vi "单参数加标流程.vi"(10 "流程类型":T4, 11 "Slave ID":T6=enum."氨氮") -> ()   [LabVIEW 2016, in "质控单元V1.lvlib"]
panel:
  in  "平行样测试数据":T1={"时间"=timestamp(0 s since 1904-01-01), "参数"="", "数据类型"="N", "第一次水样浓度值"=0.0, "第二次水样测试时间"=timestamp(0 s since 1904-01-01), "第二次水样浓度值"=0.0}
  in  "集成干预测试数据":T2={"时间"=timestamp(0 s since 1904-01-01), "参数"="", "数据类型"="N", "集成干预测试浓度值"=0.0, "集成干预前测试时间"=timestamp(0 s since 1904-01-01), "集成干预前测试浓度值"=0.0}
  out "平行样启动时间":timestamp
  out "加标模块润洗流程控制":T3=enum."排液"
  in  "获取加标回收测试数据计数":u16
  in  "获取水样测试数据计数":u16
  in  "写入加标体积重试次数":u16
  in  "加标模块加标润洗启动计数":u16
  out "加标回收启动时间":timestamp
  out "水样测试启动时间":timestamp
  out "Next State":string
  in  "仪器加标回收启动计数":u16
  in  "仪器水样测试启动计数":u16
  in  "加标模块排液启动计数":u16
  in  "加标模块加标启动计数":u16
  in  "加标模块进样启动计数":u16
  in  "加标模块水样润洗启动计数":u16
  in  "采配水启动次数计数":u16
  in  "加标回收测试时间":timestamp
  in  "水样测试时间":timestamp
  in  "质控数据":T5
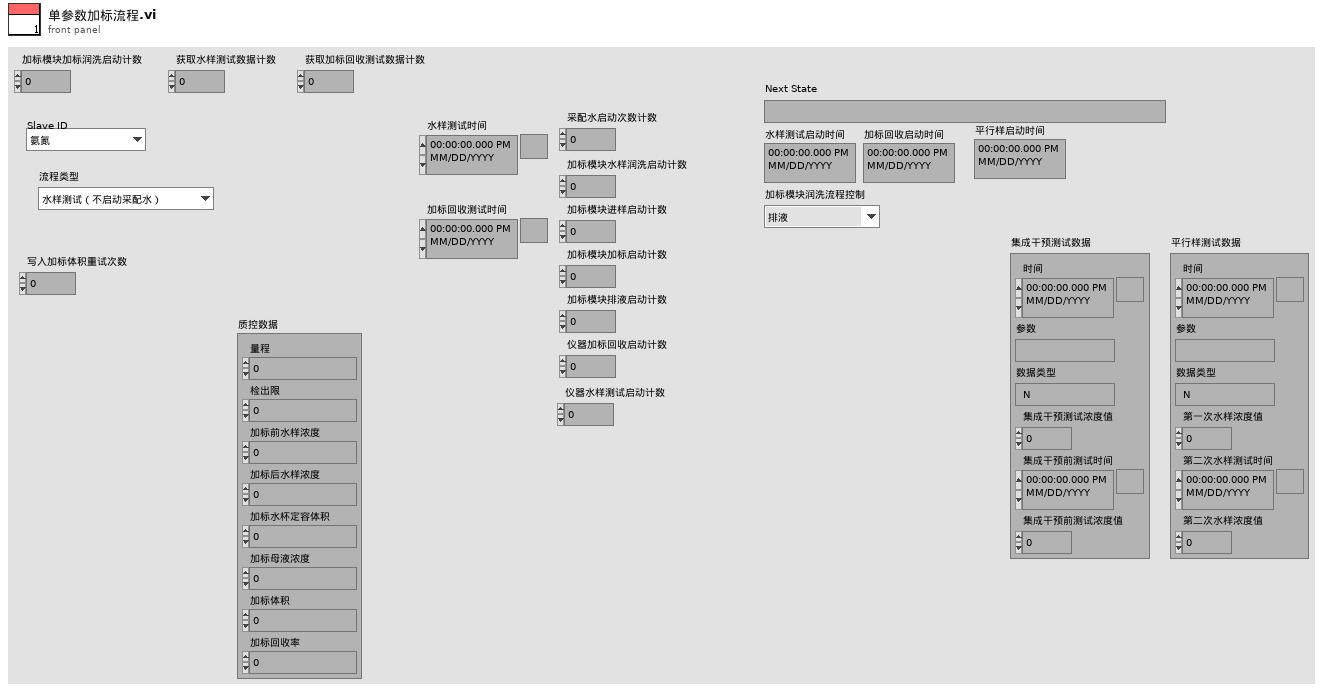
[diagram p1: front panel]
types:
  T1 = typedef "平行样测试数据字段定义.ctl" = cluster{"时间":timestamp, "参数":string, "数据类型":string, "第一次水样浓度值":dbl, "第二次水样测试时间":timestamp, "第二次水样浓度值":dbl}
  T2 = typedef "集成干预字段定义.ctl" = cluster{"时间":timestamp, "参数":string, "数据类型":string, "集成干预测试浓度值":dbl, "集成干预前测试时间":timestamp, "集成干预前测试浓度值":dbl}
  T3 = typedef "质控单元V1.lvlib/质控流程控制.ctl" = enum16{"待机", "润洗", "进样", "加标", "排液", "搅拌"}
  T4 = typedef "质控单元V1.lvlib/测试子流程.ctl" = enum16{"水样测试（不启动采配水）", "水样测试（不含采样杯）", "加标回收（润洗采样合并）", "加标回收（不启动采配水）", "平行样测试（不启动采配水）", "平行样测试（不含采样杯）", "集成干预测试（不含采样杯）"}
  T5 = cluster{"量程":dbl, "检出限":dbl, "加标前水样浓度":dbl, "加标后水样浓度":dbl, "加标水杯定容体积":dbl, "加标母液浓度":dbl, "加标体积":dbl, "加标回收率":dbl}
  T6 = typedef "质控单元V1.lvlib/质控slave id.ctl" = enum16{"null", "氨氮", "总磷", "CODMn", "CODCr", "总氮"}
  T7 = cluster{"时间":timestamp, "参数":string, "数据类型":string, "加标回收率":sgl, "加标前水样测试时间":timestamp, "加标前水样浓度值":sgl, "加标后水样浓度值":sgl, "加标母液浓度值":sgl, "加标体积":sgl, "加标水杯定容体积":sgl}
  T8 = enum16{"待机", "水样测试（全流程）", "停止", "加标回收", "水样测试（简易流程）"}
  T9 = enum16{"待机", "润洗", "采样", "沉淀", "配水", "反冲洗", "储水", "结束"}
  T10 = typedef "质控单元V1.lvlib/采配水通用流程.ctl" = enum16{"待机", "润洗", "采样", "沉淀", "配水", "反冲洗", "结束"}
  T11 = typedef "质控单元V1.lvlib/质控运行状态.ctl" = enum16{"待机", "润洗", "进样", "加标", "排液", "搅拌", "超时告警"}
  T12 = enum16{"空闲", "水样测试", "标样核查", "零点核查", "跨度核查", "空白测试", "平行样测试", "加标回收", "空白校准", "标样校准", "初始化（清洗）"}
  T13 = cluster{"时间":timestamp, "参数":string, "数据类型":string, "第一次水样浓度值":dbl, "第二次水样测试时间":timestamp, "第二次水样浓度值":dbl}
  T14 = cluster{"水样数据时间":timestamp, "水样实测值":sgl, "水样数据标识":string}
  T15 = cluster{"加标回收数据时间":timestamp, "加标回收实测值":sgl, "加标回收数据标识":string}
  T16 = typedef "质控单元V1.lvlib/质控仪器状态.ctl" = cluster{"运行状态":T11, "加标体积":sgl, "NC":dbl, "液位状态":enum16{"无感应", "有感应"}, "告警状态":enum16{"无告警", "超时告警"}}
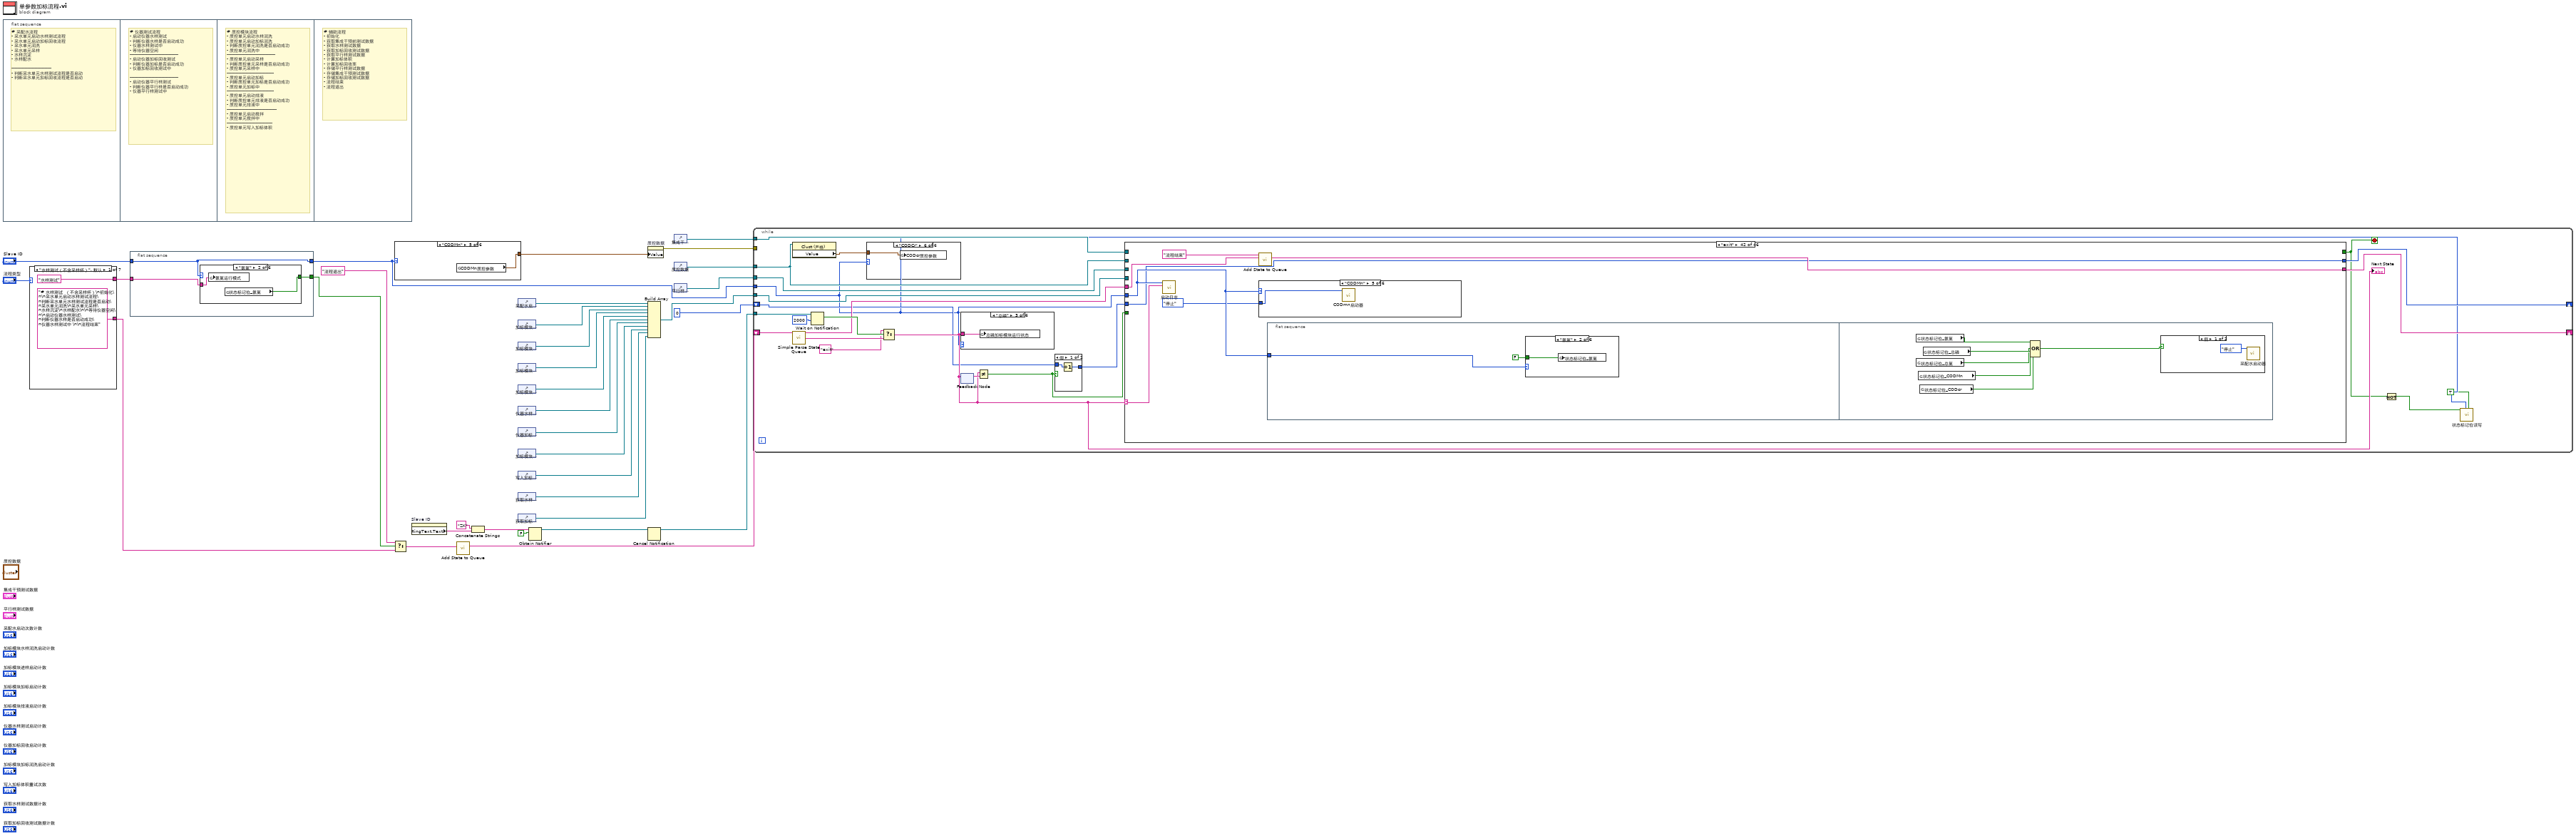
[diagram p0: block diagram]
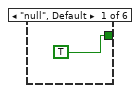
[diagram p2: hidden frame]
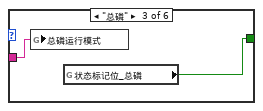
[diagram p3: hidden frame]
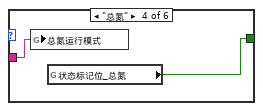
[diagram p4: hidden frame]
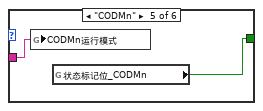
[diagram p5: hidden frame]
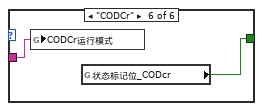
[diagram p6: hidden frame]
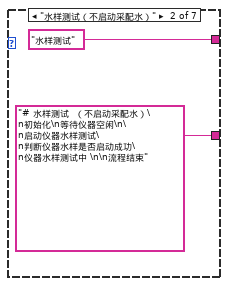
[diagram p7: hidden frame]
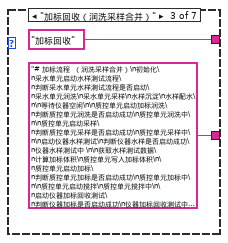
[diagram p8: hidden frame]
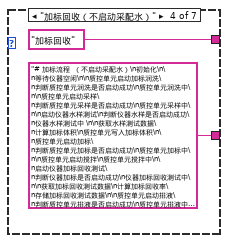
[diagram p9: hidden frame]
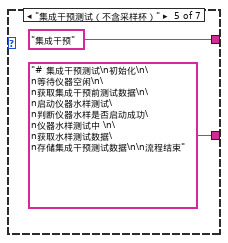
[diagram p10: hidden frame]
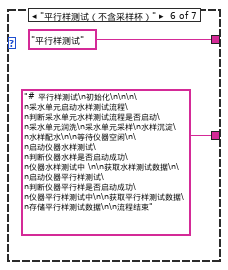
[diagram p11: hidden frame]
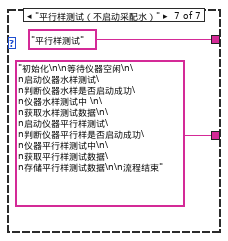
[diagram p12: hidden frame]
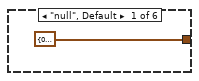
[diagram p13: hidden frame]
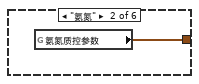
[diagram p14: hidden frame]
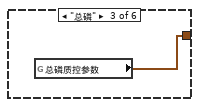
[diagram p15: hidden frame]
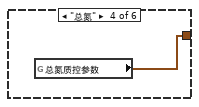
[diagram p16: hidden frame]
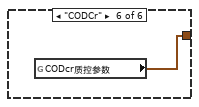
[diagram p17: hidden frame]
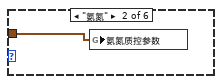
[diagram p20: hidden frame]
diagram:
  n1 = flat-sequence {
    frame #0 {
      # "# 采配水流程\n- 采水单元启动水样测试流程\n- 采水单元启动加标回收流程\n- 采水单元润洗\n- 采水单元采样 \n- 水样沉淀\n- 水样配水\n\n----------------------------\n- 判断采水单元水样测试流程是否启动\n- 判断采水单元加标回收流程是否启动"
    }
    frame #1 {
      # "# 仪器测试流程\n- 启动仪器水样测试\n- 判断仪器水样是否启动成功\n- 仪器水样测试中\n- 等待仪器空闲\n----------------------------------\n- 启动仪器加标回收测试\n- 判断仪器加标是否启动成功\n- 仪器加标回收测试中\n\n----------------------------------\n- 启动仪器平行样测试\n- 判断仪器平行样是否启动成功\n- 仪器平行样测试中"
    }
    frame #2 {
      # "# 质控模块流程\n- 质控单元启动水样润洗\n- 质控单元启动加标润洗\n- 判断质控单元润洗是否启动成功\n- 质控单元润洗中\n----------------------------------\n- 质控单元启动采样\n- 判断质控单元采样是否启动成功\n- 质控单元采样中\n---------------------------------\n- 质控单元启动加标\n- 判断质控单元加标是否启动成功\n- 质控单元加标中\n---------------------------------\n- 质控单元启动排液\n- 判断质控单元排液是否启动成功\n- 质控单元排液中\n-----------------------------------\n- 质控单元启动搅拌\n- 质控单元搅拌中\n--------------------------------\n- 质控单元写入加标体积"
    }
    frame #3 {
      # "# 辅助流程\n- 初始化\n- 获取集成干预前测试数据\n- 获取水样测试数据\n- 获取加标回收测试数据\n- 获取平行样测试数据\n- 计算加标体积\n- 计算加标回收率\n- 存储平行样测试数据\n- 存储集成干预测试数据\n- 存储加标回收测试数据 \n- 流程结束\n- 流程退出"
    }
  }
  n2 = case shown="\"水样测试（不含采样杯）\", 默认" "流程类型" {
    tunnel: ["# 水样测试  （不含采样杯）\n初始化\n\n采水单元启动水样测试流程\n判断采水单元水样测试流程是否启动\n采水单元润洗\n采水单元采样\n水样沉淀\n水样配水\n\n等待仪器空闲\n\n启动仪器水样测试\n判断仪器水样是否启动成功\n仪器水样测试中 \n\n流程结束" ("State(s) In (\"\")") "# 水样测试  （不启动采配水）\n初始化\n等待仪器空闲\n\n启动仪器水样测试\n判断仪器水样是否启动成功\n仪器水样测试中 \n\n流程结束" ("State(s) In (\"\")") "# 加标流程  （润洗采样合并）\n初始化\n采水单元启动水样测试流程\n判断采水单元水样测试流程是否启动\n采水单元润洗\n采水单元采样\n水样沉淀\n水样配水\n\n等待仪器空闲\n\n质控单元启动加标润洗\n判断质控单元润洗是否启动成功\n质控单元润洗中\n\n质控单元启动采样\n判断质控单元采样是否启动成功\n质控单元采样中\n\n启动仪器水样测试\n判断仪器水样是否启动成功\n仪器水样测试中 \n\n获取水样测试数据\n计算加标体积\n质控单元写入加标体积\n\n质控单元启动加标\n判断质控单元加标是否启动成功\n质控单元加标中\n\n质控单元启动搅拌\n质控单元搅拌中\n\n启动仪器加标回收测试\n判断仪器加标是否启动成功\n仪器加标回收测试中\n\n获取加标回收测试数据\n计算加标回收率\n存储加标回收测试数据\n\n质控单元启动排液\n判断质控单元排液是否启动成功\n质控单元排液中\n\n流程结束" ("State(s) In (\"\")") "# 加标流程  （不启动采配水）\n初始化\n\n等待仪器空闲\n\n质控单元启动加标润洗\n判断质控单元润洗是否启动成功\n质控单元润洗中\n\n质控单元启动采样\n判断质控单元采样是否启动成功\n质控单元采样中\n\n启动仪器水样测试\n判断仪器水样是否启动成功\n仪器水样测试中 \n\n获取水样测试数据\n计算加标体积\n质控单元写入加标体积\n\n质控单元启动加标\n判断质控单元加标是否启动成功\n质控单元加标中\n\n质控单元启动搅拌\n质控单元搅拌中\n\n启动仪器加标回收测试\n判断仪器加标是否启动成功\n仪器加标回收测试中\n\n获取加标回收测试数据\n计算加标回收率\n存储加标回收测试数据\n\n质控单元启动排液\n判断质控单元排液是否启动成功\n质控单元排液中\n\n流程结束" ("State(s) In (\"\")") "# 集成干预测试\n初始化\n\n等待仪器空闲\n\n获取集成干预前测试数据\n\n启动仪器水样测试\n判断仪器水样是否启动成功\n仪器水样测试中 \n\n获取水样测试数据\n存储集成干预测试数据\n\n流程结束" ("State(s) In (\"\")") "# 平行样测试\n初始化\n\n\n\n采水单元启动水样测试流程\n判断采水单元水样测试流程是否启动\n采水单元润洗\n采水单元采样\n水样沉淀\n水样配水\n\n等待仪器空闲\n\n启动仪器水样测试\n判断仪器水样是否启动成功\n仪器水样测试中 \n\n获取水样测试数据\n\n启动仪器平行样测试\n判断仪器平行样是否启动成功\n仪器平行样测试中\n\n获取平行样测试数据\n存储平行样测试数据\n\n流程结束" ("State(s) In (\"\")") "初始化\n\n等待仪器空闲\n\n启动仪器水样测试\n判断仪器水样是否启动成功\n仪器水样测试中 \n\n获取水样测试数据\n\n启动仪器平行样测试\n判断仪器平行样是否启动成功\n仪器平行样测试中\n\n获取平行样测试数据\n存储平行样测试数据\n\n流程结束" ("State(s) In (\"\")")] -> w12
    tunnel: ["水样测试" "水样测试" "加标回收" "加标回收" "集成干预" "平行样测试" "平行样测试"] -> w6
    frame "水样测试（不含采样杯）", Default {
    }
    frame "水样测试（不启动采配水）" {
    }
    frame "加标回收（润洗采样合并）" {
    }
    frame "加标回收（不启动采配水）" {
    }
    frame "集成干预测试（不含采样杯）" {
    }
    frame "平行样测试（不含采样杯）" {
    }
    frame "平行样测试（不启动采配水）" {
    }
  }
  n3 = flat-sequence {
    tunnel: [w49] -> w15
    tunnel: [w50] -> w14
    tunnel: "Slave ID" -> [w49]
    tunnel: w6 -> [w48]
    frame #0 {
      n4 = case shown="\"氨氮\"" w49 {
        tunnel: [TRUE w52 w54 w56 w58 w60] -> w50
        tunnel: w48 -> [_ w53 w55 w57 w59 w61]
        frame "null", Default {
        }
        frame "氨氮" {
          n5 = global write "ZK非断电保存全局变量.vi" "氨氮运行模式"(w53) -> ()
          n6 = global read "ZK非断电保存全局变量.vi" "状态标记位_氨氮"() -> (w52:bool)
        }
        frame "总磷" {
          n7 = global write "ZK非断电保存全局变量.vi" "总磷运行模式"(w55) -> ()
          n8 = global read "ZK非断电保存全局变量.vi" "状态标记位_总磷"() -> (w54:bool)
        }
        frame "总氮" {
          n9 = global write "ZK非断电保存全局变量.vi" "总氮运行模式"(w57) -> ()
          n10 = global read "ZK非断电保存全局变量.vi" "状态标记位_总氮"() -> (w56:bool)
        }
        frame "CODMn" {
          n11 = global write "ZK非断电保存全局变量.vi" "CODMn运行模式"(w59) -> ()
          n12 = global read "ZK非断电保存全局变量.vi" "状态标记位_CODMn"() -> (w58:bool)
        }
        frame "CODCr" {
          n13 = global write "ZK非断电保存全局变量.vi" "CODCr运行模式"(w61) -> ()
          n14 = global read "ZK非断电保存全局变量.vi" "状态标记位_CODcr"() -> (w60:bool)
        }
      }
    }
  }
  n15 = Select(t="流程退出", s=w14, f=w12) -> (s? t:f=w11:string)
  n16 = case shown="\"CODMn\"" w15 {
    tunnel: [T5 {"量程"=0.0, "检出限"=0.0, "加标前水样浓度"=0.0, "加标后水样浓度"=0.0, "加标水杯定容体积"=0.0, "加标母液浓度"=0.0, "加标体积"=0.0, "加标回收率"=0.0} ("CODcr质控参数") w63 w64 w65 w66 w67] -> w25
    frame "null", Default {
    }
    frame "氨氮" {
      n17 = global read "ZK断电保存全局变量.vi" "氨氮质控参数"() -> (w63:T5)
    }
    frame "总磷" {
      n18 = global read "ZK断电保存全局变量.vi" "总磷质控参数"() -> (w64:T5)
    }
    frame "总氮" {
      n19 = global read "ZK断电保存全局变量.vi" "总氮质控参数"() -> (w65:T5)
    }
    frame "CODMn" {
      n20 = global read "ZK断电保存全局变量.vi" "CODMn质控参数"() -> (w66:T5)
    }
    frame "CODCr" {
      n21 = global read "ZK断电保存全局变量.vi" "CODcr质控参数"() -> (w67:T5)
    }
  }
  n22 = property on="Slave ID" class="Enum (严格)"() -> ("RingText.Text"=w33:string)  [unwired: 2 in, 2 out]
  n23 = call "Add State to Queue.vi"("State(s) In (\"\")"=w11) -> ("States Out"=w27:string)  [unwired: 14 in]
  n24 = Concatenate Strings("ZK" ("字符串"), w33) -> (w31:string)
  n25 = control-ref of="采配水启动次数计数"() -> (w23:refnum<vi>)
  n26 = control-ref of="加标模块水样润洗启动计数"() -> (w22:refnum<vi>)
  n27 = control-ref of="加标模块进样启动计数"() -> (w21:refnum<vi>)
  n28 = control-ref of="加标模块加标启动计数"() -> (w20:refnum<vi>)
  n29 = control-ref of="加标模块排液启动计数"() -> (w19:refnum<vi>)
  n30 = control-ref of="仪器水样测试启动计数"() -> (w4:refnum<vi>)
  n31 = control-ref of="仪器加标回收启动计数"() -> (w5:refnum<vi>)
  n32 = control-ref of="加标模块加标润洗启动计数"() -> (w16:refnum<vi>)
  n33 = control-ref of="写入加标体积重试次数"() -> (w10:refnum<vi>)
  n34 = control-ref of="获取水样测试数据计数"() -> (w9:refnum<vi>)
  n35 = control-ref of="获取加标回收测试数据计数"() -> (w8:refnum<vi>)
  n36 = Obtain Notifier(name (unnamed)=w31, notification data type=FALSE) -> (notifier out=w29:refnum<notifier>)  [unwired: 2 in, 2 out]
  n37 = property on="质控数据" class="Clust (严格)"("Value"=w25) -> (error out=w26:errorcluster)  [unwired: 2 in, 1 out]
  n38 = Build Array(w23, w22, w21, w20, w19, w4, w5, w16, w10, w9, w8) -> (w18:refnum<vi>[])
  n39 = Cancel Notification(0:w29) -> (8:w28:refnum<notifier>)  [unwired: 1 in, 2 out]
  n40 = control-ref of="集成干预测试数据"() -> (w2:refnum<vi>)
  n41 = control-ref of="质控数据"() -> (w24:refnum<vi>)
  n42 = control-ref of="平行样测试数据"() -> (w1:refnum<vi>)
  n43 = while {
    tunnel: w28 -> [w89]
    tunnel: w15 -> [w69]
    shift-right: [w83] -> _
    shift-left: w27 -> [w90]
    tunnel: w26 -> [_]
    tunnel: w24 -> [w82]
    tunnel: w18 -> [w80]
    shift-right: [w75] -> _
    shift-left: 0 -> [w77]
    tunnel: w2 -> [w72]
    tunnel: w1 -> [w73]
    stop <- w71 stop-if-true
    n44 = property class="Clust (严格)"(reference=w82) -> ("Value"=w81:T5)  [unwired: 1 in, 2 out]
    n45 = call "Simple Parse State Queue.vi"("State Queue"=w90) -> ("Remain States"=w84:string, "Next State"=w86:string)  [unwired: 13 in]
    n46 = Wait on Notification(notifier=w89, timeout in ms (-1)=2000 ("超时毫秒(-1)")) -> (notification=w87:bool)  [unwired: 2 in, 3 out]
    n47 = case shown="\"CODCr\"" w69 {
      tunnel: w81 -> [_ w93 w94 w95 w96 w97]
      frame "null", Default {
      }
      frame "氨氮" {
        n48 = global write "ZK断电保存全局变量.vi" "氨氮质控参数"(w93) -> ()
      }
      frame "总磷" {
        n49 = global write "ZK断电保存全局变量.vi" "总磷质控参数"(w94) -> ()
      }
      frame "总氮" {
        n50 = global write "ZK断电保存全局变量.vi" "总氮质控参数"(w95) -> ()
      }
      frame "CODMn" {
        n51 = global write "ZK断电保存全局变量.vi" "CODMn质控参数"(w96) -> ()
      }
      frame "CODCr" {
        n52 = global write "ZK断电保存全局变量.vi" "CODcr质控参数"(w97) -> ()
      }
    }
    n53 = Select(t="exit" ("State(s) In (\"\")"), s=w87, f=w86) -> (s? t:f=w78:string)
    "Next State" <- w78
    n54 = case shown="\"总磷\"" w69 {
      tunnel: w78 -> [_ w98 w99 w100 w101 w102]
      frame "null", Default {
      }
      frame "氨氮" {
        n55 = global write "ZK非断电保存全局变量.vi" "氨氮加标模块运行状态"(w98) -> ()
      }
      frame "总磷" {
        n56 = global write "ZK非断电保存全局变量.vi" "总磷加标模块运行状态"(w99) -> ()
      }
      frame "总氮" {
        n57 = global write "ZK非断电保存全局变量.vi" "总氮加标模块运行状态"(w100) -> ()
      }
      frame "CODMn" {
        n58 = global write "ZK非断电保存全局变量.vi" "CODMn加标模块运行状态"(w101) -> ()
      }
      frame "CODCr" {
        n59 = global write "ZK非断电保存全局变量.vi" "CODcr加标模块运行状态"(w102) -> ()
      }
    }
    n60 = feedback-in #1(w78) -> ()
    n61 = feedback #1() -> (w79:string)  [unwired: 1 in]
    n62 = Not Equal?(x=w78, y=w79) -> (x != y?=w74:bool)
    n63 = case shown="假" w74 {
      tunnel: w77 -> [w92 _]
      tunnel: [w91 _] -> w76
      frame False {
        n64 = Increment(x=w92) -> (x+1=w91:i32)
      }
      frame True {
      }
    }
    n65 = case shown="\"exit\"" w78 {
      selector: w78 -> [_ _ w115 w140 w197 w207 w261 w312 w322 w333 w360 w377 w389 w403 _ w413 w424 w436 w457 w479 w500 w521 w543 _ w560 w573 w584 w602 w622 w634 w649 w653 w695 w733 w771 w817 _ w845 w862 w884 w902 w921 w949 w987 w1027 w1067]
      tunnel: w84 -> [w105 w108 w124 w162 w199 w233 w285 w320 w329 w347 w363 w379 w394 w407 w410 w421 w432 w451 w458 w491 w509 w529 w551 w558 w570 w582 w594 w609 w632 w644 w651 w676 w716 w754 w792 w824 w841 w854 w866 w893 w911 w923 w966 w1005 w1044 w1073]
      tunnel: [w104 w107 w123 w161 w198 w232 w284 w319 w328 w346 w362 w378 w393 w406 w409 w420 w431 w450 w472 w490 w508 w528 w550 w557 w569 w581 w593 w608 w631 w643 w650 w675 w715 w753 w791 w823 w840 w853 w865 w892 w910 w922 w965 w1004 w1043 w1072] -> w83
      tunnel: [_ _ _ _ _ _ _ _ _ _ _ _ TRUE TRUE _ _ _ _ _ _ _ _ _ _ _ _ _ _ _ _ _ _ _ _ _ _ _ _ _ _ _ _ _ _ _ _] -> w71
      tunnel: w69 -> [_ _ w114 w149 w191 w218 w272 w311 w323 w334 w361 w372 w390 w404 _ w414 w425 w435 w456 w478 w498 w518 w541 _ w561 w574 w585 w596 w623 w635 w647 w662 w702 w740 w778 w815 _ w846 w863 w885 w903 w919 w952 w991 w1030 w1066]
      tunnel: w82 -> [_ _ w120 w160 _ w231 _ w318 w327 w345 _ _ _ _ _ _ _ _ _ _ _ _ _ _ _ _ _ w607 _ _ _ _ _ _ _ _ _ _ _ _ _ _ _ _ _ _]
      tunnel: w80 -> [_ _ w111 w146 _ w209 w263 _ _ _ _ _ _ _ _ w419 w430 w440 w462 _ _ _ _ _ w563 w576 w587 w601 w626 w638 _ w667 w707 w745 w783 _ _ w849 _ w888 w906 _ w957 w997 w1036 _]
      tunnel: w76 -> [w103 w106 w110 w137 w196 w206 w260 w310 w321 w330 w359 w376 w387 w401 w408 w412 w423 w433 w454 w476 w497 w516 w540 w556 w559 w571 w583 w595 w621 w633 w646 w660 w700 w739 w776 w813 w839 w843 w864 w882 w900 w918 w951 w990 w1029 w1063]
      tunnel: [w103 w106 w110 w137 w196 w206 w260 w310 w321 w330 w359 w376 w387 w401 w408 w412 w423 w433 w454 w476 w497 w516 w540 w556 w559 w571 w583 w595 w621 w633 w646 w660 w700 w739 w776 w813 w839 w843 w864 w882 w900 w918 w951 w990 w1029 w1063] -> w75
      tunnel: w74 -> [_ _ _ _ _ _ _ _ _ _ _ _ _ _ _ _ _ _ _ w475 w496 w515 w539 _ _ _ _ _ _ _ _ w657 w701 w738 w777 w814 _ _ w860 _ _ _ w948 w988 w1026 w1064]
      tunnel: w73 -> [_ _ _ w135 _ _ w259 _ _ _ w358 _ _ _ _ _ _ _ _ _ _ _ _ _ _ _ _ _ _ _ _ _ _ _ _ _ _ _ _ _ _ _ _ _ _ _]
      tunnel: w72 -> [_ _ _ w129 w192 _ _ _ _ _ _ w375 _ _ _ _ _ _ _ _ _ _ _ _ _ _ _ _ _ _ _ _ _ _ _ _ _ _ _ _ _ _ _ _ _ _]
      frame Default {
        n66 = call "Add State to Queue.vi"("State(s) In (\"\")"=w105) -> ("States Out"=w104:string)  [unwired: 14 in]
      }
      frame "-------------------# 辅助流程 #-------------------" {
        n67 = call "Add State to Queue.vi"("State(s) In (\"\")"=w108) -> ("States Out"=w107:string)  [unwired: 14 in]
      }
      frame "初始化" {
        w116 = 0.0 ("加标前水样浓度")
        n68 = call "报警清除命令.vi"("是否启用通讯通知"=FALSE, "Slave ID"=w114) -> ()  [unwired: 9 in, 1 out]
        n69 = local write "加标回收测试时间"(timestamp(0 s since 1904-01-01) ("加标回收测试时间")) -> ()
        n70 = local write "水样测试时间"(timestamp(0 s since 1904-01-01) ("水样测试时间")) -> ()
        n71 = property class="Clust (严格)"(reference=w120) -> (reference out=w119:refnum<vi>, "Value"=w118:T5)  [unwired: 1 in, 1 out]
        n72 = for {
          tunnel: w111 -> [w126] mode=indexing
          n73 = property class="DigNum (严格)"(reference=w126, "Value"=u16 0 ("值")) -> ()  [unwired: 1 in, 2 out]
        }
        n74 = Concatenate Strings("<<" ("字符串"), w115) -> (w113:string)
        n75 = call "启动日志.vi"("日志信息"=w113, "Slave ID"=w114) -> ()  [unwired: 9 in, 1 out]
        n76 = Bundle By Name(cluster=w118, "加标前水样浓度"=w116, "加标后水样浓度"=w116, "加标体积"=w116, "加标回收率"=w116) -> (w117:T5)
        n77 = property class="Clust (严格)"(reference=w119, "Value"=w117) -> ()  [unwired: 1 in, 2 out]
        n78 = call "Add State to Queue.vi"("State(s) In (\"\")"=w124) -> ("States Out"=w123:string)  [unwired: 14 in]
      }
      frame "获取水样测试数据" {
        n79 = call "启动日志.vi"("日志信息"=w140, "Slave ID"=w149) -> ()  [unwired: 9 in, 1 out]
        n80 = property class="Clust (严格)"(reference=w129) -> (reference out=w130:refnum<vi>, "Value"=w131:T2)  [unwired: 1 in, 1 out]
        n81 = property class="Clust (严格)"(reference=w160) -> (reference out=w159:refnum<vi>, "Value"=w158:T5)  [unwired: 1 in, 1 out]
        n82 = property class="Clust (严格)"(reference=w135) -> (reference out=w136:refnum<vi>, "Value"=w134:T13)  [unwired: 1 in, 1 out]
        n83 = case shown="\"CODCr\"" w149 {
          tunnel: [sgl 0.0 ("水样实测值") w170 w174 w178 w182 w186] -> w127
          tunnel: [timestamp(0 s since 1904-01-01) ("水样数据时间") w169 w173 w177 w181 w185] -> w128
          frame "null", Default {
          }
          frame "氨氮" {
            w167 = u16 3 items=["总磷"=1, "总氮"=2, "氨氮"=3, "CODMn"=21, "CODcr"=22] ("站号")
            n84 = call-poly "获取测试数据.vi"("站号"=w167) -> ("测量数据区"=w168:T14)  [unwired: 10 in]
            n85 = Unbundle By Name(w168) -> ("水样数据时间"=w169:timestamp, "水样实测值"=w170:sgl)
          }
          frame "总磷" {
            w171 = u16 1 items=["总磷"=1, "总氮"=2, "氨氮"=3, "CODMn"=21, "CODcr"=22] ("站号")
            n86 = call-poly "获取测试数据.vi"("站号"=w171) -> ("测量数据区"=w172:T14)  [unwired: 10 in]
            n87 = Unbundle By Name(w172) -> ("水样数据时间"=w173:timestamp, "水样实测值"=w174:sgl)
          }
          frame "总氮" {
            w175 = u16 2 items=["总磷"=1, "总氮"=2, "氨氮"=3, "CODMn"=21, "CODcr"=22] ("站号")
            n88 = call-poly "获取测试数据.vi"("站号"=w175) -> ("测量数据区"=w176:T14)  [unwired: 10 in]
            n89 = Unbundle By Name(w176) -> ("水样数据时间"=w177:timestamp, "水样实测值"=w178:sgl)
          }
          frame "CODMn" {
            w179 = u16 21 items=["总磷"=1, "总氮"=2, "氨氮"=3, "CODMn"=21, "CODcr"=22] ("站号")
            n90 = call-poly "获取测试数据.vi"("站号"=w179) -> ("测量数据区"=w180:T14)  [unwired: 10 in]
            n91 = Unbundle By Name(w180) -> ("水样数据时间"=w181:timestamp, "水样实测值"=w182:sgl)
          }
          frame "CODCr" {
            w183 = u16 22 items=["总磷"=1, "总氮"=2, "氨氮"=3, "CODMn"=21, "CODcr"=22] ("站号")
            n92 = call-poly "获取测试数据.vi"("站号"=w183) -> ("测量数据区"=w184:T14)  [unwired: 10 in]
            n93 = Unbundle By Name(w184) -> ("水样数据时间"=w185:timestamp, "水样实测值"=w186:sgl)
          }
        }
        n94 = Index Array(array=w146, index=9 ("索引")) -> (element=w147:refnum<vi>)
        n95 = property class="DigNum (严格)"(reference=w147) -> (reference out=w145:refnum<vi>, "Value"=w144:u16)  [unwired: 1 in, 1 out]
        n96 = Increment(x=w144) -> (x+1=w143:u16)
        n97 = property class="DigNum (严格)"(reference=w145, "Value"=w143) -> ()  [unwired: 1 in, 2 out]
        n98 = Less Or Equal?(x=w143, y=u16 5) -> (x <= y?=w141:bool)
        n99 = Select(t=w140, s=w141, f="exit") -> (s? t:f=w138:string)
        n100 = local read "水样测试启动时间"() -> (w156:timestamp)
        n101 = local write "水样测试时间"(w128) -> ()
        n102 = Subtract(x=w128, y=w156) -> (x-y=w155:dbl)
        n103 = Bundle By Name(cluster=w158, "加标前水样浓度"=w127) -> (w157:T5)
        n104 = Bundle By Name(cluster=w131, "时间"=w128, "集成干预测试浓度值"=w127) -> (w132:T2)
        n105 = Bundle By Name(cluster=w134, "时间"=w128, "第一次水样浓度值"=w127) -> (w133:T13)
        n106 = Absolute Value(x=w155) -> (abs(x)=w154:dbl)
        n107 = property class="Clust (严格)"(reference=w159, "Value"=w157) -> ()  [unwired: 1 in, 2 out]
        n108 = property class="Clust (严格)"(reference=w130, "Value"=w132) -> ()  [unwired: 1 in, 2 out]
        n109 = property class="Clust (严格)"(reference=w136, "Value"=w133) -> ()  [unwired: 1 in, 2 out]
        n110 = Less?(x=w154, y=300.0) -> (x < y?=w150:bool)
        n111 = case shown="假" w150 {
          tunnel: w149 -> [w164 _]
          frame False {
            w163 = "获取水样数据异常" ("日志信息")
            n112 = call "启动日志.vi"("日志信息"=w163, "Slave ID"=w164) -> ()  [unwired: 9 in, 1 out]
            n113 = call "报警信息记录.vi"("报警信息"=w163, "Slave ID"=w164) -> ()  [unwired: 9 in, 1 out]
          }
          frame True {
          }
        }
        n114 = Select(t="", s=w150, f=w138) -> (s? t:f=w151:string)
        n115 = call "Add State to Queue.vi"("State(s) In Front (\"\")"=w151, "State(s) In (\"\")"=w162) -> ("States Out"=w161:string)  [unwired: 13 in]
      }
      frame "获取集成干预前测试数据" {
        n116 = call "启动日志.vi"("日志信息"=w197, "Slave ID"=w191) -> ()  [unwired: 9 in, 1 out]
        n117 = property class="Clust (严格)"(reference=w192) -> (reference out=w193:refnum<vi>, "Value"=w194:T2)  [unwired: 1 in, 1 out]
        n118 = case shown="\"CODMn\"" w191 {
          tunnel: ["" "氨氮" "总磷" "总氮" "CODMn" "CODCr"] -> w190
          frame "null", Default {
          }
          frame "氨氮" {
          }
          frame "总磷" {
          }
          frame "总氮" {
          }
          frame "CODMn" {
          }
          frame "CODCr" {
          }
        }
        n119 = call "Add State to Queue.vi"("State(s) In (\"\")"=w199) -> ("States Out"=w198:string)  [unwired: 14 in]
        n120 = call "获取最新一笔数据.vi"("table"=w190) -> ("检测值"=w189:cluster{"时间":timestamp, "检测值":dbl})  [unwired: 8 in, 2 out]
        n121 = Unbundle By Name(w189) -> ("时间"=w188:timestamp, "检测值"=w187:dbl)
        n122 = Bundle By Name(cluster=w194, "集成干预前测试时间"=w188, "集成干预前测试浓度值"=w187) -> (w195:T2)
        n123 = property class="Clust (严格)"(reference=w193, "Value"=w195) -> ()  [unwired: 1 in, 2 out]
      }
      frame "获取加标回收测试数据" {
        n124 = call "启动日志.vi"("日志信息"=w207, "Slave ID"=w218) -> ()  [unwired: 9 in, 1 out]
        n125 = property class="Clust (严格)"(reference=w231) -> (reference out=w230:refnum<vi>, "Value"=w229:T5)  [unwired: 1 in, 1 out]
        n126 = case shown="\"CODCr\"" w218 {
          tunnel: [sgl 0.0 ("水样实测值") w241 w245 w249 w253 w257] -> w227
          tunnel: [timestamp(0 s since 1904-01-01) ("加标回收数据时间") w240 w244 w248 w252 w256] -> w224
          frame "null", Default {
          }
          frame "氨氮" {
            w238 = u16 3 items=["总磷"=1, "总氮"=2, "氨氮"=3, "CODMn"=21, "CODcr"=22] ("站号")
            n127 = call-poly "获取测试数据.vi"("站号"=w238) -> ("测量数据区"=w239:T15)  [unwired: 10 in]
            n128 = Unbundle By Name(w239) -> ("加标回收数据时间"=w240:timestamp, "加标回收实测值"=w241:sgl)
          }
          frame "总磷" {
            w242 = u16 1 items=["总磷"=1, "总氮"=2, "氨氮"=3, "CODMn"=21, "CODcr"=22] ("站号")
            n129 = call-poly "获取测试数据.vi"("站号"=w242) -> ("测量数据区"=w243:T15)  [unwired: 10 in]
            n130 = Unbundle By Name(w243) -> ("加标回收数据时间"=w244:timestamp, "加标回收实测值"=w245:sgl)
          }
          frame "总氮" {
            w246 = u16 2 items=["总磷"=1, "总氮"=2, "氨氮"=3, "CODMn"=21, "CODcr"=22] ("站号")
            n131 = call-poly "获取测试数据.vi"("站号"=w246) -> ("测量数据区"=w247:T15)  [unwired: 10 in]
            n132 = Unbundle By Name(w247) -> ("加标回收数据时间"=w248:timestamp, "加标回收实测值"=w249:sgl)
          }
          frame "CODMn" {
            w250 = u16 21 items=["总磷"=1, "总氮"=2, "氨氮"=3, "CODMn"=21, "CODcr"=22] ("站号")
            n133 = call-poly "获取测试数据.vi"("站号"=w250) -> ("测量数据区"=w251:T15)  [unwired: 10 in]
            n134 = Unbundle By Name(w251) -> ("加标回收数据时间"=w252:timestamp, "加标回收实测值"=w253:sgl)
          }
          frame "CODCr" {
            w254 = u16 22 items=["总磷"=1, "总氮"=2, "氨氮"=3, "CODMn"=21, "CODcr"=22] ("站号")
            n135 = call-poly "获取测试数据.vi"("站号"=w254) -> ("测量数据区"=w255:T15)  [unwired: 10 in]
            n136 = Unbundle By Name(w255) -> ("加标回收数据时间"=w256:timestamp, "加标回收实测值"=w257:sgl)
          }
        }
        n137 = Index Array(array=w209, index=10 ("索引")) -> (element=w217:refnum<vi>)
        n138 = property class="DigNum (严格)"(reference=w217) -> (reference out=w215:refnum<vi>, "Value"=w214:u16)  [unwired: 1 in, 1 out]
        n139 = Increment(x=w214) -> (x+1=w213:u16)
        n140 = property class="DigNum (严格)"(reference=w215, "Value"=w213) -> ()  [unwired: 1 in, 2 out]
        n141 = Less Or Equal?(x=w213, y=u16 5) -> (x <= y?=w211:bool)
        n142 = Select(t=w207, s=w211, f="exit") -> (s? t:f=w208:string)
        n143 = local read "加标回收启动时间"() -> (w225:timestamp)
        n144 = local write "加标回收测试时间"(w224) -> ()
        n145 = Subtract(x=w224, y=w225) -> (x-y=w223:dbl)
        n146 = Bundle By Name(cluster=w229, "加标后水样浓度"=w227) -> (w228:T5)
        n147 = Absolute Value(x=w223) -> (abs(x)=w220:dbl)
        n148 = property class="Clust (严格)"(reference=w230, "Value"=w228) -> ()  [unwired: 1 in, 2 out]
        n149 = Less?(x=w220, y=300.0) -> (x < y?=w219:bool)
        n150 = case shown="假" w219 {
          tunnel: w218 -> [w235 _]
          frame False {
            w234 = "获取加标数据异常" ("日志信息")
            n151 = call "启动日志.vi"("日志信息"=w234, "Slave ID"=w235) -> ()  [unwired: 9 in, 1 out]
            n152 = call "报警信息记录.vi"("报警信息"=w234, "Slave ID"=w235) -> ()  [unwired: 9 in, 1 out]
          }
          frame True {
          }
        }
        n153 = Select(t="", s=w219, f=w208) -> (s? t:f=w221:string)
        n154 = call "Add State to Queue.vi"("State(s) In Front (\"\")"=w221, "State(s) In (\"\")"=w233) -> ("States Out"=w232:string)  [unwired: 13 in]
      }
      frame "获取平行样测试数据" {
        n155 = call "启动日志.vi"("日志信息"=w261, "Slave ID"=w272) -> ()  [unwired: 9 in, 1 out]
        n156 = property class="Clust (严格)"(reference=w259) -> (reference out=w283:refnum<vi>, "Value"=w282:T13)  [unwired: 1 in, 1 out]
        n157 = case shown="\"CODCr\"" w272 {
          tunnel: [sgl 0.0 ("水样实测值") w293 w297 w301 w305 w309] -> w280
          tunnel: [timestamp(0 s since 1904-01-01) ("加标回收数据时间") w292 w296 w300 w304 w308] -> w258
          frame "null", Default {
          }
          frame "氨氮" {
            w290 = u16 3 items=["总磷"=1, "总氮"=2, "氨氮"=3, "CODMn"=21, "CODcr"=22] ("站号")
            n158 = call-poly "获取测试数据.vi"("站号"=w290) -> ("测量数据区"=w291:T14)  [unwired: 10 in]
            n159 = Unbundle By Name(w291) -> ("水样数据时间"=w292:timestamp, "水样实测值"=w293:sgl)
          }
          frame "总磷" {
            w294 = u16 1 items=["总磷"=1, "总氮"=2, "氨氮"=3, "CODMn"=21, "CODcr"=22] ("站号")
            n160 = call-poly "获取测试数据.vi"("站号"=w294) -> ("测量数据区"=w295:T14)  [unwired: 10 in]
            n161 = Unbundle By Name(w295) -> ("水样数据时间"=w296:timestamp, "水样实测值"=w297:sgl)
          }
          frame "总氮" {
            w298 = u16 2 items=["总磷"=1, "总氮"=2, "氨氮"=3, "CODMn"=21, "CODcr"=22] ("站号")
            n162 = call-poly "获取测试数据.vi"("站号"=w298) -> ("测量数据区"=w299:T14)  [unwired: 10 in]
            n163 = Unbundle By Name(w299) -> ("水样数据时间"=w300:timestamp, "水样实测值"=w301:sgl)
          }
          frame "CODMn" {
            w302 = u16 21 items=["总磷"=1, "总氮"=2, "氨氮"=3, "CODMn"=21, "CODcr"=22] ("站号")
            n164 = call-poly "获取测试数据.vi"("站号"=w302) -> ("测量数据区"=w303:T14)  [unwired: 10 in]
            n165 = Unbundle By Name(w303) -> ("水样数据时间"=w304:timestamp, "水样实测值"=w305:sgl)
          }
          frame "CODCr" {
            w306 = u16 22 items=["总磷"=1, "总氮"=2, "氨氮"=3, "CODMn"=21, "CODcr"=22] ("站号")
            n166 = call-poly "获取测试数据.vi"("站号"=w306) -> ("测量数据区"=w307:T14)  [unwired: 10 in]
            n167 = Unbundle By Name(w307) -> ("水样数据时间"=w308:timestamp, "水样实测值"=w309:sgl)
          }
        }
        n168 = Index Array(array=w263, index=10 ("索引")) -> (element=w271:refnum<vi>)
        n169 = property class="DigNum (严格)"(reference=w271) -> (reference out=w269:refnum<vi>, "Value"=w268:u16)  [unwired: 1 in, 1 out]
        n170 = Increment(x=w268) -> (x+1=w267:u16)
        n171 = property class="DigNum (严格)"(reference=w269, "Value"=w267) -> ()  [unwired: 1 in, 2 out]
        n172 = Less Or Equal?(x=w267, y=u16 5) -> (x <= y?=w265:bool)
        n173 = Select(t=w261, s=w265, f="exit") -> (s? t:f=w262:string)
        n174 = Bundle By Name(cluster=w282, "第二次水样测试时间"=w258, "第二次水样浓度值"=w280) -> (w281:T13)
        n175 = local read "平行样启动时间"() -> (w278:timestamp)
        n176 = Subtract(x=w258, y=w278) -> (x-y=w277:dbl)
        n177 = property class="Clust (严格)"(reference=w283, "Value"=w281) -> ()  [unwired: 1 in, 2 out]
        n178 = Absolute Value(x=w277) -> (abs(x)=w274:dbl)
        n179 = Less?(x=w274, y=300.0) -> (x < y?=w273:bool)
        n180 = case shown="假" w273 {
          tunnel: w272 -> [w287 _]
          frame False {
            w286 = "获取平行样数据异常" ("日志信息")
            n181 = call "启动日志.vi"("日志信息"=w286, "Slave ID"=w287) -> ()  [unwired: 9 in, 1 out]
            n182 = call "报警信息记录.vi"("报警信息"=w286, "Slave ID"=w287) -> ()  [unwired: 9 in, 1 out]
          }
          frame True {
          }
        }
        n183 = Select(t="", s=w273, f=w262) -> (s? t:f=w275:string)
        n184 = call "Add State to Queue.vi"("State(s) In Front (\"\")"=w275, "State(s) In (\"\")"=w285) -> ("States Out"=w284:string)  [unwired: 13 in]
      }
      frame "计算加标体积" {
        n185 = call "启动日志.vi"("日志信息"=w312, "Slave ID"=w311) -> ()  [unwired: 9 in, 1 out]
        n186 = property class="Clust (严格)"(reference=w318) -> (reference out=w317:refnum<vi>, "Value"=w316:T5)  [unwired: 1 in, 1 out]
        n187 = call "加标回收率计算.vi"("参数"=w316) -> ("参数 out"=w315:T5)  [unwired: 9 in, 1 out]
        n188 = Bundle By Name(cluster=w315, "加标回收率"=0.0) -> (w314:T5)
        n189 = property class="Clust (严格)"(reference=w317, "Value"=w314) -> ()  [unwired: 1 in, 2 out]
        n190 = call "Add State to Queue.vi"("State(s) In (\"\")"=w320) -> ("States Out"=w319:string)  [unwired: 14 in]
      }
      frame "计算加标回收率" {
        n191 = call "启动日志.vi"("日志信息"=w322, "Slave ID"=w323) -> ()  [unwired: 9 in, 1 out]
        n192 = property class="Clust (严格)"(reference=w327) -> (reference out=w326:refnum<vi>, "Value"=w325:T5)  [unwired: 1 in, 1 out]
        n193 = call "加标回收率计算.vi"("参数"=w325) -> ("参数 out"=w324:T5)  [unwired: 9 in, 1 out]
        n194 = property class="Clust (严格)"(reference=w326, "Value"=w324) -> ()  [unwired: 1 in, 2 out]
        n195 = call "Add State to Queue.vi"("State(s) In (\"\")"=w329) -> ("States Out"=w328:string)  [unwired: 14 in]
      }
      frame "存储加标回收测试数据" {
        n196 = call "启动日志.vi"("日志信息"=w333, "Slave ID"=w334) -> ()  [unwired: 9 in, 1 out]
        n197 = property class="Clust (严格)"(reference=w345) -> ("Value"=w342:T5)  [unwired: 1 in, 2 out]
        n198 = case shown="\"总氮\"" w334 {
          tunnel: ["" "氨氮加标回收率" "总磷加标回收率" "总氮加标回收率" "CODMn加标回收率" "CODCr加标回收率"] -> w335
          frame "null", Default {
          }
          frame "氨氮" {
          }
          frame "总磷" {
          }
          frame "总氮" {
          }
          frame "CODMn" {
          }
          frame "CODCr" {
          }
        }
        n199 = Unbundle By Name(w342) -> ("加标前水样浓度"=w341:dbl, "加标后水样浓度"=w340:dbl, "加标母液浓度"=w339:dbl, "加标体积"=w338:dbl, "加标水杯定容体积"=w337:dbl, "加标回收率"=w336:dbl)
        n200 = call "Add State to Queue.vi"("State(s) In (\"\")"=w347) -> ("States Out"=w346:string)  [unwired: 14 in]
        n201 = Bundle By Name(cluster=T7 {"时间"=timestamp(0 s since 1904-01-01), "参数"="", "数据类型"="N", "加标回收率"=0.0, "加标前水样测试时间"=timestamp(0 s since 1904-01-01), "加标前水样浓度值"=0.0, "加标后水样浓度值"=0.0, "加标母液浓度值"=0.0, "加标体积"=0.0, "加标水杯定容体积"=0.0} ("data in"), "时间"="加标回收测试时间", "参数"=w335, "加标前水样测试时间"="水样测试时间", "加标前水样浓度值"=w341, "加标后水样浓度值"=w340, "加标母液浓度值"=w339, "加标体积"=w338, "加标水杯定容体积"=w337, "加标回收率"=w336) -> (w331:T7)
        n202 = call "加标回收数据插入.vi"("data in"=w331) -> ()  [unwired: 10 in, 1 out]
      }
      frame "存储平行样测试数据" {
        n203 = call "启动日志.vi"("日志信息"=w360, "Slave ID"=w361) -> ()  [unwired: 9 in, 1 out]
        n204 = property class="Clust (严格)"(reference=w358) -> (reference out=w356:refnum<vi>, "Value"=w357:T13)  [unwired: 1 in, 1 out]
        n205 = case shown="\"CODMn\"" w361 {
          tunnel: ["" "氨氮" "总磷" "总氮" "CODMn" "CODCr"] -> w354
          frame "null", Default {
          }
          frame "氨氮" {
          }
          frame "总磷" {
          }
          frame "总氮" {
          }
          frame "CODMn" {
          }
          frame "CODCr" {
          }
        }
        n206 = call "Add State to Queue.vi"("State(s) In (\"\")"=w363) -> ("States Out"=w362:string)  [unwired: 14 in]
        n207 = Bundle By Name(cluster=w357, "参数"=w354) -> (w355:T13)
        n208 = property class="Clust (严格)"(reference=w356, "Value"=w355) -> ()  [unwired: 1 in, 2 out]
        n209 = call "平行样数据插入.vi"("平行样测试数据"=w355) -> ()  [unwired: 10 in, 1 out]
      }
      frame "存储集成干预测试数据" {
        n210 = call "启动日志.vi"("日志信息"=w377, "Slave ID"=w372) -> ()  [unwired: 9 in, 1 out]
        n211 = property class="Clust (严格)"(reference=w375) -> (reference out=w373:refnum<vi>, "Value"=w374:T2)  [unwired: 1 in, 1 out]
        n212 = case shown="\"CODMn\"" w372 {
          tunnel: ["" "氨氮" "总磷" "总氮" "CODMn" "CODCr"] -> w371
          frame "null", Default {
          }
          frame "氨氮" {
          }
          frame "总磷" {
          }
          frame "总氮" {
          }
          frame "CODMn" {
          }
          frame "CODCr" {
          }
        }
        n213 = call "Add State to Queue.vi"("State(s) In (\"\")"=w379) -> ("States Out"=w378:string)  [unwired: 14 in]
        n214 = Bundle By Name(cluster=w374, "参数"=w371) -> (w370:T2)
        n215 = property class="Clust (严格)"(reference=w373, "Value"=w370) -> ()  [unwired: 1 in, 2 out]
        n216 = call "集成干预数据插入.vi"("集成干预测试数据"=w370) -> ()  [unwired: 10 in, 1 out]
      }
      frame "流程结束" {
        n217 = case shown="\"CODCr\"" w390 {
          tunnel: "空闲" -> [_ w395 w396 w397 w398 w399]
          frame "null", Default {
          }
          frame "氨氮" {
            n218 = global write "ZK非断电保存全局变量.vi" "氨氮加标模块运行状态"(w395) -> ()
          }
          frame "总磷" {
            n219 = global write "ZK非断电保存全局变量.vi" "总磷加标模块运行状态"(w396) -> ()
          }
          frame "总氮" {
            n220 = global write "ZK非断电保存全局变量.vi" "总氮加标模块运行状态"(w397) -> ()
          }
          frame "CODMn" {
            n221 = global write "ZK非断电保存全局变量.vi" "CODMn加标模块运行状态"(w398) -> ()
          }
          frame "CODCr" {
            n222 = global write "ZK非断电保存全局变量.vi" "CODcr加标模块运行状态"(w399) -> ()
          }
        }
        n223 = Concatenate Strings(w389, ">>" ("字符串")) -> (w388:string)
        n224 = call "启动日志.vi"("日志信息"=w388, "Slave ID"=w390) -> ()  [unwired: 9 in, 1 out]
        n225 = call "Add State to Queue.vi"("State(s) In (\"\")"=w394) -> ("States Out"=w393:string)  [unwired: 14 in]
      }
      frame "流程退出" {
        n226 = Concatenate Strings(w403, ">>" ("字符串")) -> (w402:string)
        n227 = call "启动日志.vi"("日志信息"=w402, "Slave ID"=w404) -> ()  [unwired: 9 in, 1 out]
        n228 = call "Add State to Queue.vi"("State(s) In (\"\")"=w407) -> ("States Out"=w406:string)  [unwired: 14 in]
      }
      frame "-------------------# 采配水流程 #-------------------" {
        n229 = call "Add State to Queue.vi"("State(s) In (\"\")"=w410) -> ("States Out"=w409:string)  [unwired: 14 in]
      }
      frame "采水单元启动水样测试流程" {
        n230 = call "启动日志.vi"("日志信息"=w413, "Slave ID"=w414) -> ()  [unwired: 9 in, 1 out]
        n231 = call "采配水启动器.vi"("启动/停止命令"=T8."水样测试（全流程）") -> ()  [unwired: 10 in, 1 out]
        n232 = Index Array(array=w419) -> (element=w418:refnum<vi>)  [unwired: 1 in]
        n233 = property class="DigNum (严格)"(reference=w418) -> (reference out=w417:refnum<vi>, "Value"=w416:u16)  [unwired: 1 in, 1 out]
        n234 = Increment(x=w416) -> (x+1=w415:u16)
        n235 = property class="DigNum (严格)"(reference=w417, "Value"=w415) -> ()  [unwired: 1 in, 2 out]
        n236 = call "Add State to Queue.vi"("State(s) In (\"\")"=w421) -> ("States Out"=w420:string)  [unwired: 14 in]
      }
      frame "采水单元启动加标回收流程" {
        n237 = call "启动日志.vi"("日志信息"=w424, "Slave ID"=w425) -> ()  [unwired: 9 in, 1 out]
        n238 = call "采配水启动器.vi"("启动/停止命令"=T8."加标回收") -> ()  [unwired: 10 in, 1 out]
        n239 = Index Array(array=w430) -> (element=w429:refnum<vi>)  [unwired: 1 in]
        n240 = property class="DigNum (严格)"(reference=w429) -> (reference out=w428:refnum<vi>, "Value"=w427:u16)  [unwired: 1 in, 1 out]
        n241 = Increment(x=w427) -> (x+1=w426:u16)
        n242 = property class="DigNum (严格)"(reference=w428, "Value"=w426) -> ()  [unwired: 1 in, 2 out]
        n243 = call "Add State to Queue.vi"("State(s) In (\"\")"=w432) -> ("States Out"=w431:string)  [unwired: 14 in]
      }
      frame "判断采水单元水样测试流程是否启动" {
        n244 = call "获取采配水运行状态.vi"() -> ("运行流程"=w449:T10)  [unwired: 10 in, 1 out]
        n245 = call "启动日志.vi"("日志信息"=w436, "Slave ID"=w435) -> ()  [unwired: 9 in, 1 out]
        n246 = Equal?(x=T9."待机" ("运行流程"), y=w449) -> (x = y?=w448:bool)
        n247 = Index Array(array=w440, index=0 ("索引")) -> (element=w439:refnum<vi>)
        n248 = property class="DigNum (严格)"(reference=w439) -> ("Value"=w438:u16)  [unwired: 1 in, 2 out]
        n249 = Greater Or Equal?(x=w438, y=u16 5) -> (x >= y?=w434:bool)
        n250 = Select(t="采水单元启动水样测试流程\n判断采水单元水样测试流程是否启动" ("State(s) In (\"\")"), s=w448, f="") -> (s? t:f=w443:string)
        n251 = case shown="真" w434 {
          tunnel: w435 -> [_ w453]
          frame False {
          }
          frame True {
            w452 = "采水单元启动失败" ("日志信息")
            n252 = call "启动日志.vi"("日志信息"=w452, "Slave ID"=w453) -> ()  [unwired: 9 in, 1 out]
            n253 = call "报警信息记录.vi"("报警信息"=w452, "Slave ID"=w453) -> ()  [unwired: 9 in, 1 out]
          }
        }
        n254 = Select(t="流程结束" ("State(s) In (\"\")"), s=w434, f=w443) -> (s? t:f=w442:string)
        n255 = call "Add State to Queue.vi"("State(s) In Front (\"\")"=w442, "State(s) In (\"\")"=w451) -> ("States Out"=w450:string)  [unwired: 13 in]
      }
      frame "判断采水单元加标回收流程是否启动" {
        n256 = call "获取采配水运行状态.vi"() -> ("运行流程"=w471:T10)  [unwired: 10 in, 1 out]
        n257 = call "启动日志.vi"("日志信息"=w457, "Slave ID"=w456) -> ()  [unwired: 9 in, 1 out]
        n258 = Equal?(x=T9."待机" ("运行流程"), y=w471) -> (x = y?=w470:bool)
        n259 = Index Array(array=w462, index=0 ("索引")) -> (element=w461:refnum<vi>)
        n260 = property class="DigNum (严格)"(reference=w461) -> ("Value"=w460:u16)  [unwired: 1 in, 2 out]
        n261 = Greater Or Equal?(x=w460, y=u16 5) -> (x >= y?=w455:bool)
        n262 = Select(t="采水单元启动加标回收流程\n判断采水单元加标回收流程是否启动" ("State(s) In (\"\")"), s=w470, f="") -> (s? t:f=w465:string)
        n263 = case shown="真" w455 {
          tunnel: w456 -> [_ w474]
          frame False {
          }
          frame True {
            w473 = "采水单元启动失败" ("日志信息")
            n264 = call "启动日志.vi"("日志信息"=w473, "Slave ID"=w474) -> ()  [unwired: 9 in, 1 out]
            n265 = call "报警信息记录.vi"("报警信息"=w473, "Slave ID"=w474) -> ()  [unwired: 9 in, 1 out]
          }
        }
        n266 = Select(t="流程结束" ("State(s) In (\"\")"), s=w455, f=w465) -> (s? t:f=w464:string)
        n267 = call "Add State to Queue.vi"("State(s) In Front (\"\")"=w464, "State(s) In (\"\")"=w458) -> ("States Out"=w472:string)  [unwired: 13 in]
      }
      frame "采水单元润洗" {
        n268 = call "获取采配水运行状态.vi"() -> ("运行流程"=w485:T10)  [unwired: 10 in, 1 out]
        n269 = Equal To 0?(x=w485) -> (x = 0?=w477:bool)
        n270 = Less?(x=w485, y=T9."采样" ("运行流程")) -> (x < y?=w488:bool)
        n271 = Greater?(x=w485, y=T9."待机" ("运行流程")) -> (0:w489:bool)
        n272 = case shown="真" w475 {
          tunnel: w478 -> [_ w495]
          tunnel: w479 -> [_ w494]
          frame False {
          }
          frame True {
            n273 = call "启动日志.vi"("日志信息"=w494, "Slave ID"=w495) -> ()  [unwired: 9 in, 1 out]
          }
        }
        n274 = And(x=w488, y=w489) -> (x .and. y?=w487:bool)
        n275 = case shown="真" w477 {
          tunnel: w478 -> [_ w493]
          frame False {
          }
          frame True {
            w492 = "采水单元流程中断" ("日志信息")
            n276 = call "启动日志.vi"("日志信息"=w492, "Slave ID"=w493) -> ()  [unwired: 9 in, 1 out]
            n277 = call "报警信息记录.vi"("报警信息"=w492, "Slave ID"=w493) -> ()  [unwired: 9 in, 1 out]
          }
        }
        n278 = Select(t=w479, s=w487, f="") -> (s? t:f=w483:string)
        n279 = Select(t="流程结束" ("State(s) In (\"\")"), s=w477, f=w483) -> (s? t:f=w482:string)
        n280 = call "Add State to Queue.vi"("State(s) In Front (\"\")"=w482, "State(s) In (\"\")"=w491) -> ("States Out"=w490:string)  [unwired: 13 in]
      }
      frame "采水单元采样" {
        n281 = call "获取采配水运行状态.vi"() -> ("运行流程"=w502:T10)  [unwired: 10 in, 1 out]
        n282 = Equal To 0?(x=w502) -> (x = 0?=w499:bool)
        n283 = Equal?(x=T9."采样" ("运行流程"), y=w502) -> (x = y?=w501:bool)
        n284 = case shown="真" w496 {
          tunnel: w498 -> [_ w513]
          tunnel: w500 -> [_ w512]
          frame False {
          }
          frame True {
            n285 = call "启动日志.vi"("日志信息"=w512, "Slave ID"=w513) -> ()  [unwired: 9 in, 1 out]
          }
        }
        n286 = case shown="真" w499 {
          tunnel: w498 -> [_ w511]
          frame False {
          }
          frame True {
            w510 = "采水单元流程中断" ("日志信息")
            n287 = call "启动日志.vi"("日志信息"=w510, "Slave ID"=w511) -> ()  [unwired: 9 in, 1 out]
            n288 = call "报警信息记录.vi"("报警信息"=w510, "Slave ID"=w511) -> ()  [unwired: 9 in, 1 out]
          }
        }
        n289 = Select(t=w500, s=w501, f="") -> (s? t:f=w505:string)
        n290 = Select(t="流程结束" ("State(s) In (\"\")"), s=w499, f=w505) -> (s? t:f=w504:string)
        n291 = call "Add State to Queue.vi"("State(s) In Front (\"\")"=w504, "State(s) In (\"\")"=w509) -> ("States Out"=w508:string)  [unwired: 13 in]
      }
      frame "水样沉淀" {
        n292 = global read "系统交互.vi" "站点类型"() -> (w519:enum16{"一体站", "固定站", "浮船", "一体站V1-V3"})
        n293 = case shown="\"浮船\"" w519 {
          tunnel: [w533 _ _] -> w520
          tunnel: w515 -> [w532 _ _]
          frame "一体站", Default {
            n294 = case shown="真" w532 {
              tunnel: [_ w534] -> w533
              frame False {
              }
              frame True {
                n295 = call "质控模块润洗OK命令.vi"("质控润洗OK"=TRUE) -> ("error out"=w534:errorcluster)  [unwired: 10 in]
              }
            }
          }
          frame "固定站" {
          }
          frame "浮船" {
          }
        }
        n296 = case shown="真" w515 {
          tunnel: w518 -> [_ w537]
          tunnel: w521 -> [_ w536]
          frame False {
          }
          frame True {
            n297 = call "启动日志.vi"("日志信息"=w536, "Slave ID"=w537) -> ()  [unwired: 9 in, 1 out]
          }
        }
        n298 = call "获取采配水运行状态.vi"("error in (no error)"=w520) -> ("运行流程"=w525:T10)  [unwired: 9 in, 1 out]
        n299 = Equal To 0?(x=w525) -> (x = 0?=w517:bool)
        n300 = Equal?(x=采配水通用流程."沉淀" ("运行流程"), y=w525) -> (x = y?=w527:bool)
        n301 = case shown="真" w517 {
          tunnel: w518 -> [_ w531]
          frame False {
          }
          frame True {
            w530 = "采水单元流程中断" ("日志信息")
            n302 = call "启动日志.vi"("日志信息"=w530, "Slave ID"=w531) -> ()  [unwired: 9 in, 1 out]
            n303 = call "报警信息记录.vi"("报警信息"=w530, "Slave ID"=w531) -> ()  [unwired: 9 in, 1 out]
          }
        }
        n304 = Select(t=w521, s=w527, f="") -> (s? t:f=w523:string)
        n305 = Select(t="流程结束" ("State(s) In (\"\")"), s=w517, f=w523) -> (s? t:f=w522:string)
        n306 = call "Add State to Queue.vi"("State(s) In Front (\"\")"=w522, "State(s) In (\"\")"=w529) -> ("States Out"=w528:string)  [unwired: 13 in]
      }
      frame "水样配水" {
        n307 = call "获取采配水运行状态.vi"() -> ("运行流程"=w548:T10)  [unwired: 10 in, 1 out]
        n308 = Equal To 0?(x=w548) -> (x = 0?=w542:bool)
        n309 = Equal?(x=采配水通用流程."配水" ("运行流程"), y=w548) -> (x = y?=w549:bool)
        n310 = case shown="真" w539 {
          tunnel: w541 -> [_ w555]
          tunnel: w543 -> [_ w554]
          frame False {
          }
          frame True {
            n311 = call "启动日志.vi"("日志信息"=w554, "Slave ID"=w555) -> ()  [unwired: 9 in, 1 out]
          }
        }
        n312 = case shown="真" w542 {
          tunnel: w541 -> [_ w553]
          frame False {
          }
          frame True {
            w552 = "采水单元流程中断" ("日志信息")
            n313 = call "启动日志.vi"("日志信息"=w552, "Slave ID"=w553) -> ()  [unwired: 9 in, 1 out]
            n314 = call "报警信息记录.vi"("报警信息"=w552, "Slave ID"=w553) -> ()  [unwired: 9 in, 1 out]
          }
        }
        n315 = Select(t="", s=w549, f=w543) -> (s? t:f=w546:string)
        n316 = Select(t="流程结束" ("State(s) In (\"\")"), s=w542, f=w546) -> (s? t:f=w545:string)
        n317 = call "Add State to Queue.vi"("State(s) In Front (\"\")"=w545, "State(s) In (\"\")"=w551) -> ("States Out"=w550:string)  [unwired: 13 in]
      }
      frame "-------------------# 质控模块流程 #-------------------" {
        n318 = call "Add State to Queue.vi"("State(s) In (\"\")"=w558) -> ("States Out"=w557:string)  [unwired: 14 in]
      }
      frame "质控单元启动水样润洗" {
        w568 = 质控流程控制."润洗" ("流程控制")
        n319 = call "启动日志.vi"("日志信息"=w560, "Slave ID"=w561) -> ()  [unwired: 9 in, 1 out]
        n320 = call "单步流程命令.vi"("流程控制"=w568, "Slave ID"=w561) -> ()  [unwired: 9 in, 1 out]
        n321 = Index Array(array=w563, index=1 ("索引")) -> (element=w567:refnum<vi>)
        n322 = property class="DigNum (严格)"(reference=w567) -> (reference out=w566:refnum<vi>, "Value"=w565:u16)  [unwired: 1 in, 1 out]
        n323 = Increment(x=w565) -> (x+1=w564:u16)
        n324 = property class="DigNum (严格)"(reference=w566, "Value"=w564) -> ()  [unwired: 1 in, 2 out]
        n325 = call "Add State to Queue.vi"("State(s) In (\"\")"=w570) -> ("States Out"=w569:string)  [unwired: 14 in]
        "加标模块润洗流程控制" <- w568
      }
      frame "质控单元启动加标润洗" {
        w572 = 质控流程控制."润洗" ("流程控制")
        n326 = call "启动日志.vi"("日志信息"=w573, "Slave ID"=w574) -> ()  [unwired: 9 in, 1 out]
        n327 = call "单步流程命令.vi"("流程控制"=w572, "Slave ID"=w574) -> ()  [unwired: 9 in, 1 out]
        n328 = local write "加标模块润洗流程控制"(w572) -> ()
        n329 = Index Array(array=w576, index=7 ("索引")) -> (element=w580:refnum<vi>)
        n330 = property class="DigNum (严格)"(reference=w580) -> (reference out=w579:refnum<vi>, "Value"=w578:u16)  [unwired: 1 in, 1 out]
        n331 = Increment(x=w578) -> (x+1=w577:u16)
        n332 = property class="DigNum (严格)"(reference=w579, "Value"=w577) -> ()  [unwired: 1 in, 2 out]
        n333 = call "Add State to Queue.vi"("State(s) In (\"\")"=w582) -> ("States Out"=w581:string)  [unwired: 14 in]
      }
      frame "质控单元启动采样" {
        n334 = call "启动日志.vi"("日志信息"=w584, "Slave ID"=w585) -> ()  [unwired: 9 in, 1 out]
        n335 = call "单步流程命令.vi"("流程控制"=质控流程控制."润洗", "Slave ID"=w585) -> ()  [unwired: 9 in, 1 out]
        n336 = Index Array(array=w587, index=2 ("索引")) -> (element=w591:refnum<vi>)
        n337 = property class="DigNum (严格)"(reference=w591) -> (reference out=w590:refnum<vi>, "Value"=w589:u16)  [unwired: 1 in, 1 out]
        n338 = Increment(x=w589) -> (x+1=w588:u16)
        n339 = property class="DigNum (严格)"(reference=w590, "Value"=w588) -> ()  [unwired: 1 in, 2 out]
        n340 = call "Add State to Queue.vi"("State(s) In (\"\")"=w594) -> ("States Out"=w593:string)  [unwired: 14 in]
      }
      frame "质控单元写入加标体积" {
        n341 = call "启动日志.vi"("日志信息"=w602, "Slave ID"=w596) -> ()  [unwired: 9 in, 1 out]
        n342 = property class="Clust (严格)"(reference=w607) -> ("Value"=w606:T5)  [unwired: 1 in, 2 out]
        n343 = Index Array(array=w601, index=8 ("索引")) -> (element=w599:refnum<vi>)
        n344 = Unbundle By Name(w606) -> ("加标体积"=w605:dbl)
        n345 = property class="DigNum (严格)"(reference=w599) -> (reference out=w597:refnum<vi>, "Value"=w598:u16)  [unwired: 1 in, 1 out]
        n346 = call "加标体积写入.vi"("加标体积"=w605, "Slave ID"=w596) -> ("error out"=w604:errorcluster)  [unwired: 9 in]
        n347 = case shown="错误" w604 {
          tunnel: [_ w612] -> w603
          tunnel: w602 -> [_ w614]
          tunnel: w598 -> [_ w616]
          tunnel: w597 -> [_ w618]
          tunnel: w596 -> [_ w610]
          frame No Error {
          }
          frame Error {
            n348 = Increment(x=w616) -> (x+1=w617:u16)
            n349 = Greater Or Equal?(x=w616, y=u16 5) -> (x >= y?=w611:bool)
            n350 = property class="DigNum (严格)"(reference=w618, "Value"=w617) -> ()  [unwired: 1 in, 2 out]
            n351 = case shown="真" w611 {
              tunnel: w610 -> [_ w620]
              frame False {
              }
              frame True {
                w619 = "加标体积写入异常" ("报警信息")
                n352 = call "启动日志.vi"("日志信息"=w619, "Slave ID"=w620) -> ()  [unwired: 9 in, 1 out]
                n353 = call "报警信息记录.vi"("报警信息"=w619, "Slave ID"=w620) -> ()  [unwired: 9 in, 1 out]
              }
            }
            n354 = Select(t="流程结束", s=w611, f=w614) -> (s? t:f=w612:string)
          }
        }
        n355 = call "Add State to Queue.vi"("State(s) In Front (\"\")"=w603, "State(s) In (\"\")"=w609) -> ("States Out"=w608:string)  [unwired: 13 in]
      }
      frame "质控单元启动加标" {
        n356 = call "启动日志.vi"("日志信息"=w622, "Slave ID"=w623) -> ()  [unwired: 9 in, 1 out]
        n357 = call "单步流程命令.vi"("流程控制"=质控流程控制."加标", "Slave ID"=w623) -> ()  [unwired: 9 in, 1 out]
        n358 = Index Array(array=w626, index=3 ("索引")) -> (element=w625:refnum<vi>)
        n359 = property class="DigNum (严格)"(reference=w625) -> (reference out=w629:refnum<vi>, "Value"=w628:u16)  [unwired: 1 in, 1 out]
        n360 = Increment(x=w628) -> (x+1=w627:u16)
        n361 = property class="DigNum (严格)"(reference=w629, "Value"=w627) -> ()  [unwired: 1 in, 2 out]
        n362 = call "Add State to Queue.vi"("State(s) In (\"\")"=w632) -> ("States Out"=w631:string)  [unwired: 14 in]
      }
      frame "质控单元启动排液" {
        n363 = call "启动日志.vi"("日志信息"=w634, "Slave ID"=w635) -> ()  [unwired: 9 in, 1 out]
        n364 = call "单步流程命令.vi"("流程控制"=质控流程控制."排液", "Slave ID"=w635) -> ()  [unwired: 9 in, 1 out]
        n365 = Index Array(array=w638, index=4 ("索引")) -> (element=w637:refnum<vi>)
        n366 = property class="DigNum (严格)"(reference=w637) -> (reference out=w641:refnum<vi>, "Value"=w640:u16)  [unwired: 1 in, 1 out]
        n367 = Increment(x=w640) -> (x+1=w639:u16)
        n368 = property class="DigNum (严格)"(reference=w641, "Value"=w639) -> ()  [unwired: 1 in, 2 out]
        n369 = call "Add State to Queue.vi"("State(s) In (\"\")"=w644) -> ("States Out"=w643:string)  [unwired: 14 in]
      }
      frame "质控单元启动搅拌" {
        n370 = call "启动日志.vi"("日志信息"=w649, "Slave ID"=w647) -> ()  [unwired: 9 in, 1 out]
        n371 = call "单步流程命令.vi"("是否启用通讯通知"=FALSE, "流程控制"=质控流程控制."搅拌", "Slave ID"=w647) -> ()  [unwired: 8 in, 1 out]
        n372 = call "Add State to Queue.vi"("State(s) In (\"\")"=w651) -> ("States Out"=w650:string)  [unwired: 14 in]
      }
      frame "判断质控单元润洗是否启动成功" {
        n373 = local read "加标模块润洗流程控制"() -> (w661:T3)
        n374 = case shown="真" w657 {
          tunnel: w653 -> [_ w678]
          tunnel: w662 -> [_ w677]
          frame False {
          }
          frame True {
            n375 = call "启动日志.vi"("日志信息"=w678, "Slave ID"=w677) -> ()  [unwired: 9 in, 1 out]
          }
        }
        n376 = case shown="\"null\", 默认" w662 {
          tunnel: [_ w683 w685 w687 w689 w691] -> w674
          frame "null", Default {
          }
          frame "氨氮" {
            n377 = global read "ZK非断电保存全局变量.vi" "氨氮质控仪器状态"() -> (w684:T16)
            n378 = Unbundle By Name(w684) -> ("运行状态"=w683:T11)
          }
          frame "总磷" {
            n379 = global read "ZK非断电保存全局变量.vi" "总磷质控仪器状态"() -> (w686:T16)
            n380 = Unbundle By Name(w686) -> ("运行状态"=w685:T11)
          }
          frame "总氮" {
            n381 = global read "ZK非断电保存全局变量.vi" "总氮质控仪器状态"() -> (w688:T16)
            n382 = Unbundle By Name(w688) -> ("运行状态"=w687:T11)
          }
          frame "CODMn" {
            n383 = global read "ZK非断电保存全局变量.vi" "CODMn质控仪器状态"() -> (w690:T16)
            n384 = Unbundle By Name(w690) -> ("运行状态"=w689:T11)
          }
          frame "CODCr" {
            n385 = global read "ZK非断电保存全局变量.vi" "CODCr质控仪器状态"() -> (w692:T16)
            n386 = Unbundle By Name(w692) -> ("运行状态"=w691:T11)
          }
        }
        n387 = case shown="\"排液\", 默认" w661 {
          tunnel: ["质控单元启动水样润洗\n判断质控单元润洗是否启动成功" ("State(s) In (\"\")") "质控单元启动加标润洗\n判断质控单元润洗是否启动成功" ("State(s) In (\"\")")] -> w655
          frame "排液", Default {
          }
          frame "搅拌" {
          }
        }
        n388 = Index Array(array=w667, index=1 ("索引")) -> (element=w666:refnum<vi>)
        n389 = Greater Or Equal?(x=w660, y=10) -> (x >= y?=w656:bool)
        n390 = property class="DigNum (严格)"(reference=w666) -> ("Value"=w665:u16)  [unwired: 1 in, 2 out]
        n391 = Greater Or Equal?(x=w665, y=u16 5) -> (x >= y?=w663:bool)
        n392 = Select(t=w655, s=w656, f=w653) -> (s? t:f=w654:string)
        n393 = case shown="真" w663 {
          tunnel: w662 -> [_ w682]
          frame False {
          }
          frame True {
            w681 = "质控单元润洗启动失败" ("日志信息")
            n394 = call "启动日志.vi"("日志信息"=w681, "Slave ID"=w682) -> ()  [unwired: 9 in, 1 out]
            n395 = call "报警信息记录.vi"("报警信息"=w681, "Slave ID"=w682) -> ()  [unwired: 9 in, 1 out]
          }
        }
        n396 = Not Equal?(x=w674, y=质控运行状态."待机" ("运行状态")) -> (x != y?=w673:bool)
        n397 = And(x=w656, y=w673) -> (x .and. y?=w658:bool)
        n398 = Select(t="", s=w658, f=w654) -> (s? t:f=w671:string)
        n399 = Select(t="流程结束" ("State(s) In (\"\")"), s=w663, f=w671) -> (s? t:f=w669:string)
        n400 = call "Add State to Queue.vi"("State(s) In Front (\"\")"=w669, "State(s) In (\"\")"=w676) -> ("States Out"=w675:string)  [unwired: 13 in]
      }
      frame "判断质控单元采样是否启动成功" {
        n401 = case shown="真" w701 {
          tunnel: w695 -> [_ w718]
          tunnel: w702 -> [_ w717]
          frame False {
          }
          frame True {
            n402 = call "启动日志.vi"("日志信息"=w718, "Slave ID"=w717) -> ()  [unwired: 9 in, 1 out]
          }
        }
        n403 = case shown="\"null\", 默认" w702 {
          tunnel: [_ w721 w723 w725 w727 w729] -> w714
          frame "null", Default {
          }
          frame "氨氮" {
            n404 = global read "ZK非断电保存全局变量.vi" "氨氮质控仪器状态"() -> (w722:T16)
            n405 = Unbundle By Name(w722) -> ("运行状态"=w721:T11)
          }
          frame "总磷" {
            n406 = global read "ZK非断电保存全局变量.vi" "总磷质控仪器状态"() -> (w724:T16)
            n407 = Unbundle By Name(w724) -> ("运行状态"=w723:T11)
          }
          frame "总氮" {
            n408 = global read "ZK非断电保存全局变量.vi" "总氮质控仪器状态"() -> (w726:T16)
            n409 = Unbundle By Name(w726) -> ("运行状态"=w725:T11)
          }
          frame "CODMn" {
            n410 = global read "ZK非断电保存全局变量.vi" "CODMn质控仪器状态"() -> (w728:T16)
            n411 = Unbundle By Name(w728) -> ("运行状态"=w727:T11)
          }
          frame "CODCr" {
            n412 = global read "ZK非断电保存全局变量.vi" "CODCr质控仪器状态"() -> (w730:T16)
            n413 = Unbundle By Name(w730) -> ("运行状态"=w729:T11)
          }
        }
        n414 = Index Array(array=w707, index=2 ("索引")) -> (element=w706:refnum<vi>)
        n415 = Greater Or Equal?(x=w700, y=10) -> (x >= y?=w697:bool)
        n416 = property class="DigNum (严格)"(reference=w706) -> ("Value"=w705:u16)  [unwired: 1 in, 2 out]
        n417 = Select(t="质控单元启动采样\n判断质控单元采样是否启动成功" ("State(s) In (\"\")"), s=w697, f=w695) -> (s? t:f=w694:string)
        n418 = Greater Or Equal?(x=w705, y=u16 5) -> (x >= y?=w703:bool)
        n419 = case shown="真" w703 {
          tunnel: w702 -> [_ w720]
          frame False {
          }
          frame True {
            w719 = "质控单元采样启动失败" ("日志信息")
            n420 = call "启动日志.vi"("日志信息"=w719, "Slave ID"=w720) -> ()  [unwired: 9 in, 1 out]
            n421 = call "报警信息记录.vi"("报警信息"=w719, "Slave ID"=w720) -> ()  [unwired: 9 in, 1 out]
          }
        }
        n422 = Not Equal?(x=w714, y=质控运行状态."待机" ("运行状态")) -> (x != y?=w713:bool)
        n423 = And(x=w697, y=w713) -> (x .and. y?=w698:bool)
        n424 = Select(t="", s=w698, f=w694) -> (s? t:f=w711:string)
        n425 = Select(t="流程结束" ("State(s) In (\"\")"), s=w703, f=w711) -> (s? t:f=w709:string)
        n426 = call "Add State to Queue.vi"("State(s) In Front (\"\")"=w709, "State(s) In (\"\")"=w716) -> ("States Out"=w715:string)  [unwired: 13 in]
      }
      frame "判断质控单元加标是否启动成功" {
        n427 = case shown="真" w738 {
          tunnel: w733 -> [_ w756]
          tunnel: w740 -> [_ w755]
          frame False {
          }
          frame True {
            n428 = call "启动日志.vi"("日志信息"=w756, "Slave ID"=w755) -> ()  [unwired: 9 in, 1 out]
          }
        }
        n429 = case shown="\"null\", 默认" w740 {
          tunnel: [_ w759 w761 w763 w765 w767] -> w752
          frame "null", Default {
          }
          frame "氨氮" {
            n430 = global read "ZK非断电保存全局变量.vi" "氨氮质控仪器状态"() -> (w760:T16)
            n431 = Unbundle By Name(w760) -> ("运行状态"=w759:T11)
          }
          frame "总磷" {
            n432 = global read "ZK非断电保存全局变量.vi" "总磷质控仪器状态"() -> (w762:T16)
            n433 = Unbundle By Name(w762) -> ("运行状态"=w761:T11)
          }
          frame "总氮" {
            n434 = global read "ZK非断电保存全局变量.vi" "总氮质控仪器状态"() -> (w764:T16)
            n435 = Unbundle By Name(w764) -> ("运行状态"=w763:T11)
          }
          frame "CODMn" {
            n436 = global read "ZK非断电保存全局变量.vi" "CODMn质控仪器状态"() -> (w766:T16)
            n437 = Unbundle By Name(w766) -> ("运行状态"=w765:T11)
          }
          frame "CODCr" {
            n438 = global read "ZK非断电保存全局变量.vi" "CODCr质控仪器状态"() -> (w768:T16)
            n439 = Unbundle By Name(w768) -> ("运行状态"=w767:T11)
          }
        }
        n440 = Index Array(array=w745, index=3 ("索引")) -> (element=w744:refnum<vi>)
        n441 = Greater Or Equal?(x=w739, y=10) -> (x >= y?=w735:bool)
        n442 = property class="DigNum (严格)"(reference=w744) -> ("Value"=w743:u16)  [unwired: 1 in, 2 out]
        n443 = Select(t="质控单元启动加标\n判断质控单元加标是否启动成功" ("State(s) In (\"\")"), s=w735, f=w733) -> (s? t:f=w732:string)
        n444 = Greater Or Equal?(x=w743, y=u16 5) -> (x >= y?=w741:bool)
        n445 = case shown="真" w741 {
          tunnel: w740 -> [_ w758]
          frame False {
          }
          frame True {
            w757 = "质控单元加标启动失败" ("日志信息")
            n446 = call "启动日志.vi"("日志信息"=w757, "Slave ID"=w758) -> ()  [unwired: 9 in, 1 out]
            n447 = call "报警信息记录.vi"("报警信息"=w757, "Slave ID"=w758) -> ()  [unwired: 9 in, 1 out]
          }
        }
        n448 = Not Equal?(x=w752, y=质控运行状态."待机" ("运行状态")) -> (x != y?=w751:bool)
        n449 = And(x=w735, y=w751) -> (x .and. y?=w736:bool)
        n450 = Select(t="", s=w736, f=w732) -> (s? t:f=w749:string)
        n451 = Select(t="流程结束" ("State(s) In (\"\")"), s=w741, f=w749) -> (s? t:f=w747:string)
        n452 = call "Add State to Queue.vi"("State(s) In Front (\"\")"=w747, "State(s) In (\"\")"=w754) -> ("States Out"=w753:string)  [unwired: 13 in]
      }
      frame "判断质控单元排液是否启动成功" {
        n453 = case shown="真" w777 {
          tunnel: w771 -> [_ w794]
          tunnel: w778 -> [_ w793]
          frame False {
          }
          frame True {
            n454 = call "启动日志.vi"("日志信息"=w794, "Slave ID"=w793) -> ()  [unwired: 9 in, 1 out]
          }
        }
        n455 = case shown="\"氨氮\"" w778 {
          tunnel: [_ w797 w799 w801 w803 w805] -> w790
          frame "null", Default {
          }
          frame "氨氮" {
            n456 = global read "ZK非断电保存全局变量.vi" "氨氮质控仪器状态"() -> (w798:T16)
            n457 = Unbundle By Name(w798) -> ("运行状态"=w797:T11)
          }
          frame "总磷" {
            n458 = global read "ZK非断电保存全局变量.vi" "总磷质控仪器状态"() -> (w800:T16)
            n459 = Unbundle By Name(w800) -> ("运行状态"=w799:T11)
          }
          frame "总氮" {
            n460 = global read "ZK非断电保存全局变量.vi" "总氮质控仪器状态"() -> (w802:T16)
            n461 = Unbundle By Name(w802) -> ("运行状态"=w801:T11)
          }
          frame "CODMn" {
            n462 = global read "ZK非断电保存全局变量.vi" "CODMn质控仪器状态"() -> (w804:T16)
            n463 = Unbundle By Name(w804) -> ("运行状态"=w803:T11)
          }
          frame "CODCr" {
            n464 = global read "ZK非断电保存全局变量.vi" "CODCr质控仪器状态"() -> (w806:T16)
            n465 = Unbundle By Name(w806) -> ("运行状态"=w805:T11)
          }
        }
        n466 = Index Array(array=w783, index=4 ("索引")) -> (element=w782:refnum<vi>)
        n467 = Greater Or Equal?(x=w776, y=10) -> (x >= y?=w773:bool)
        n468 = property class="DigNum (严格)"(reference=w782) -> ("Value"=w781:u16)  [unwired: 1 in, 2 out]
        n469 = Select(t="质控单元启动排液\n判断质控单元排液是否启动成功" ("State(s) In (\"\")"), s=w773, f=w771) -> (s? t:f=w770:string)
        n470 = Greater Or Equal?(x=w781, y=u16 5) -> (x >= y?=w779:bool)
        n471 = case shown="真" w779 {
          tunnel: w778 -> [_ w796]
          frame False {
          }
          frame True {
            w795 = "质控单元排液启动失败" ("日志信息")
            n472 = call "启动日志.vi"("日志信息"=w795, "Slave ID"=w796) -> ()  [unwired: 9 in, 1 out]
            n473 = call "报警信息记录.vi"("报警信息"=w795, "Slave ID"=w796) -> ()  [unwired: 9 in, 1 out]
          }
        }
        n474 = Not Equal?(x=w790, y=质控运行状态."待机" ("运行状态")) -> (x != y?=w789:bool)
        n475 = And(x=w773, y=w789) -> (x .and. y?=w774:bool)
        n476 = Select(t="", s=w774, f=w770) -> (s? t:f=w787:string)
        n477 = Select(t="流程结束" ("State(s) In (\"\")"), s=w779, f=w787) -> (s? t:f=w785:string)
        n478 = call "Add State to Queue.vi"("State(s) In Front (\"\")"=w785, "State(s) In (\"\")"=w792) -> ("States Out"=w791:string)  [unwired: 13 in]
      }
      frame "质控单元采样中", "质控单元加标中", "质控单元搅拌中", "质控单元排液中", "质控单元润洗中" {
        n479 = case shown="\"null\", 默认" w815 {
          tunnel: [_ w829 w831 w833 w835 w837] -> w816
          frame "null", Default {
          }
          frame "氨氮" {
            n480 = global read "ZK非断电保存全局变量.vi" "氨氮质控仪器状态"() -> (w830:T16)
            n481 = Unbundle By Name(w830) -> ("运行状态"=w829:T11)
          }
          frame "总磷" {
            n482 = global read "ZK非断电保存全局变量.vi" "总磷质控仪器状态"() -> (w832:T16)
            n483 = Unbundle By Name(w832) -> ("运行状态"=w831:T11)
          }
          frame "总氮" {
            n484 = global read "ZK非断电保存全局变量.vi" "总氮质控仪器状态"() -> (w834:T16)
            n485 = Unbundle By Name(w834) -> ("运行状态"=w833:T11)
          }
          frame "CODMn" {
            n486 = global read "ZK非断电保存全局变量.vi" "CODMn质控仪器状态"() -> (w836:T16)
            n487 = Unbundle By Name(w836) -> ("运行状态"=w835:T11)
          }
          frame "CODCr" {
            n488 = global read "ZK非断电保存全局变量.vi" "CODCr质控仪器状态"() -> (w838:T16)
            n489 = Unbundle By Name(w838) -> ("运行状态"=w837:T11)
          }
        }
        n490 = case shown="真" w814 {
          tunnel: w815 -> [_ w828]
          tunnel: w817 -> [_ w827]
          frame False {
          }
          frame True {
            n491 = call "启动日志.vi"("日志信息"=w827, "Slave ID"=w828) -> ()  [unwired: 9 in, 1 out]
          }
        }
        n492 = Greater Or Equal?(x=w813, y=15) -> (x >= y?=w810:bool)
        n493 = Equal?(x=w816, y=质控运行状态."超时告警" ("运行状态")) -> (x = y?=w807:bool)
        n494 = Equal?(x=w816, y=质控运行状态."待机" ("运行状态")) -> (x = y?=w822:bool)
        n495 = And(x=w810, y=w822) -> (x .and. y?=w811:bool)
        n496 = case shown="真" w807 {
          tunnel: w815 -> [_ w826]
          frame False {
          }
          frame True {
            w825 = "质控单元流程中断" ("日志信息")
            n497 = call "启动日志.vi"("日志信息"=w825, "Slave ID"=w826) -> ()  [unwired: 9 in, 1 out]
            n498 = call "报警信息记录.vi"("报警信息"=w825, "Slave ID"=w826) -> ()  [unwired: 9 in, 1 out]
          }
        }
        n499 = Select(t="", s=w811, f=w817) -> (s? t:f=w820:string)
        n500 = Select(t="流程结束" ("State(s) In (\"\")"), s=w807, f=w820) -> (s? t:f=w818:string)
        n501 = call "Add State to Queue.vi"("State(s) In Front (\"\")"=w818, "State(s) In (\"\")"=w824) -> ("States Out"=w823:string)  [unwired: 13 in]
      }
      frame "-------------------# 仪器测试流程 #-------------------" {
        n502 = call "Add State to Queue.vi"("State(s) In (\"\")"=w841) -> ("States Out"=w840:string)  [unwired: 14 in]
      }
      frame "启动仪器水样测试" {
        n503 = Get Date/Time In Seconds() -> (seconds since 1Jan1904=→"水样测试启动时间":timestamp)
        n504 = call "启动日志.vi"("日志信息"=w845, "Slave ID"=w846) -> ()  [unwired: 9 in, 1 out]
        n505 = case shown="\"总氮\"" w846 {
          tunnel: enum16{"水样测试", "平行样测试", "加标回收", "停止"}."水样测试" ("控制命令") -> [_ w855 w856 w857 w858 w859]
          frame "null", Default {
          }
          frame "氨氮" {
            n506 = call "氨氮启动器.vi"("控制命令"=w855) -> ()  [unwired: 11 in]
          }
          frame "总磷" {
            n507 = call "总磷启动器.vi"("控制命令"=w856) -> ()  [unwired: 11 in]
          }
          frame "总氮" {
            n508 = call "总氮启动器.vi"("控制命令"=w857) -> ()  [unwired: 11 in]
          }
          frame "CODMn" {
            n509 = call "CODmn启动器.vi"("控制命令"=w858) -> ()  [unwired: 11 in]
          }
          frame "CODCr" {
            n510 = call "CODcr启动器.vi"("控制命令"=w859) -> ()  [unwired: 11 in]
          }
        }
        n511 = Index Array(array=w849, index=5 ("索引")) -> (element=w848:refnum<vi>)
        n512 = property class="DigNum (严格)"(reference=w848) -> (reference out=w852:refnum<vi>, "Value"=w851:u16)  [unwired: 1 in, 1 out]
        n513 = Increment(x=w851) -> (x+1=w850:u16)
        n514 = property class="DigNum (严格)"(reference=w852, "Value"=w850) -> ()  [unwired: 1 in, 2 out]
        n515 = call "Add State to Queue.vi"("State(s) In (\"\")"=w854) -> ("States Out"=w853:string)  [unwired: 14 in]
      }
      frame "等待仪器空闲" {
        n516 = case shown="真" w860 {
          tunnel: w863 -> [_ w880]
          tunnel: w862 -> [_ w879]
          frame False {
          }
          frame True {
            n517 = call "启动日志.vi"("日志信息"=w879, "Slave ID"=w880) -> ()  [unwired: 9 in, 1 out]
          }
        }
        n518 = case shown="\"总磷\"" w863 {
          tunnel: w862 -> [_ w871]
          tunnel: [_ w870] -> w861
          frame "null", Default {
          }
          frame "总磷" {
            n519 = global read "系统交互.vi" "总磷总氮类型"() -> (w867:enum16{"单模块", "总磷总氮二合一模块", "氨氮总磷二合一模块"})
            n520 = Not Equal?(x=w867, y=enum16{"单模块", "总磷总氮二合一模块", "氨氮总磷二合一模块"}."单模块") -> (x != y?=w868:bool)
            n521 = case shown="真" w868 {
              tunnel: w871 -> [_ w876]
              tunnel: [_ w875] -> w870
              tunnel: w867 -> [_ w873]
              frame False {
              }
              frame True {
                n522 = case shown="\"总磷总氮二合一模块\"" w873 {
                  tunnel: [_ w877 w878] -> w872
                  frame "单模块", Default {
                  }
                  frame "总磷总氮二合一模块" {
                    n523 = global read "ZK非断电保存全局变量.vi" "状态标记位_总氮"() -> (w877:bool)
                  }
                  frame "氨氮总磷二合一模块" {
                    n524 = global read "ZK非断电保存全局变量.vi" "状态标记位_氨氮"() -> (w878:bool)
                  }
                }
                n525 = Select(t=w876, s=w872, f="") -> (s? t:f=w875:string)
              }
            }
          }
        }
        n526 = call "Add State to Queue.vi"("State(s) In Front (\"\")"=w861, "State(s) In (\"\")"=w866) -> ("States Out"=w865:string)  [unwired: 13 in]
      }
      frame "启动仪器加标回收测试" {
        n527 = Get Date/Time In Seconds() -> (seconds since 1Jan1904=→"加标回收启动时间":timestamp)
        n528 = call "启动日志.vi"("日志信息"=w884, "Slave ID"=w885) -> ()  [unwired: 9 in, 1 out]
        n529 = case shown="\"CODMn\"" w885 {
          tunnel: enum16{"水样测试", "平行样测试", "加标回收", "停止"}."加标回收" ("控制命令") -> [_ w894 w895 w896 w897 w898]
          frame "null", Default {
          }
          frame "氨氮" {
            n530 = call "氨氮启动器.vi"("控制命令"=w894) -> ()  [unwired: 11 in]
          }
          frame "总磷" {
            n531 = call "总磷启动器.vi"("控制命令"=w895) -> ()  [unwired: 11 in]
          }
          frame "总氮" {
            n532 = call "总氮启动器.vi"("控制命令"=w896) -> ()  [unwired: 11 in]
          }
          frame "CODMn" {
            n533 = call "CODmn启动器.vi"("控制命令"=w897) -> ()  [unwired: 11 in]
          }
          frame "CODCr" {
            n534 = call "CODcr启动器.vi"("控制命令"=w898) -> ()  [unwired: 11 in]
          }
        }
        n535 = Index Array(array=w888, index=6 ("索引")) -> (element=w887:refnum<vi>)
        n536 = property class="DigNum (严格)"(reference=w887) -> (reference out=w891:refnum<vi>, "Value"=w890:u16)  [unwired: 1 in, 1 out]
        n537 = Increment(x=w890) -> (x+1=w889:u16)
        n538 = property class="DigNum (严格)"(reference=w891, "Value"=w889) -> ()  [unwired: 1 in, 2 out]
        n539 = call "Add State to Queue.vi"("State(s) In (\"\")"=w893) -> ("States Out"=w892:string)  [unwired: 14 in]
      }
      frame "启动仪器平行样测试" {
        n540 = Get Date/Time In Seconds() -> (seconds since 1Jan1904=→"平行样启动时间":timestamp)
        n541 = call "启动日志.vi"("日志信息"=w902, "Slave ID"=w903) -> ()  [unwired: 9 in, 1 out]
        n542 = case shown="\"总磷\"" w903 {
          tunnel: enum16{"水样测试", "平行样测试", "加标回收", "停止"}."平行样测试" ("控制命令") -> [_ w912 w913 w914 w915 w916]
          frame "null", Default {
          }
          frame "氨氮" {
            n543 = call "氨氮启动器.vi"("控制命令"=w912) -> ()  [unwired: 11 in]
          }
          frame "总磷" {
            n544 = call "总磷启动器.vi"("控制命令"=w913) -> ()  [unwired: 11 in]
          }
          frame "总氮" {
            n545 = call "总氮启动器.vi"("控制命令"=w914) -> ()  [unwired: 11 in]
          }
          frame "CODMn" {
            n546 = call "CODmn启动器.vi"("控制命令"=w915) -> ()  [unwired: 11 in]
          }
          frame "CODCr" {
            n547 = call "CODcr启动器.vi"("控制命令"=w916) -> ()  [unwired: 11 in]
          }
        }
        n548 = Index Array(array=w906, index=6 ("索引")) -> (element=w905:refnum<vi>)
        n549 = property class="DigNum (严格)"(reference=w905) -> (reference out=w909:refnum<vi>, "Value"=w908:u16)  [unwired: 1 in, 1 out]
        n550 = Increment(x=w908) -> (x+1=w907:u16)
        n551 = property class="DigNum (严格)"(reference=w909, "Value"=w907) -> ()  [unwired: 1 in, 2 out]
        n552 = call "Add State to Queue.vi"("State(s) In (\"\")"=w911) -> ("States Out"=w910:string)  [unwired: 14 in]
      }
      frame "exit" {
        n553 = call "启动日志.vi"("日志信息"=w921, "Slave ID"=w919) -> ()  [unwired: 9 in, 1 out]
        n554 = call "Add State to Queue.vi"("State(s) In Front (\"\")"="流程结束" ("State(s) In Front (\"\")"), "State(s) In (\"\")"=w923) -> ("States Out"=w922:string)  [unwired: 13 in]
        n555 = case shown="\"CODMn\"" w919 {
          tunnel: enum16{"水样测试", "平行样测试", "加标回收", "停止"}."停止" ("控制命令") -> [_ w938 w939 w940 w941 w942]
          frame "null", Default {
          }
          frame "氨氮" {
            n556 = call "氨氮启动器.vi"("控制命令"=w938) -> ()  [unwired: 11 in]
          }
          frame "总磷" {
            n557 = call "总磷启动器.vi"("控制命令"=w939) -> ()  [unwired: 11 in]
          }
          frame "总氮" {
            n558 = call "总氮启动器.vi"("控制命令"=w940) -> ()  [unwired: 11 in]
          }
          frame "CODMn" {
            n559 = call "CODmn启动器.vi"("控制命令"=w941) -> ()  [unwired: 11 in]
          }
          frame "CODCr" {
            n560 = call "CODcr启动器.vi"("控制命令"=w942) -> ()  [unwired: 11 in]
          }
        }
        n561 = flat-sequence {
          tunnel: w919 -> [w925]
          frame #0 {
            n562 = case shown="\"氨氮\"" w925 {
              tunnel: FALSE -> [_ w926 w927 w928 w929 w930]
              frame "null", Default {
              }
              frame "氨氮" {
                n563 = global write "ZK非断电保存全局变量.vi" "状态标记位_氨氮"(w926) -> ()
              }
              frame "总磷" {
                n564 = global write "ZK非断电保存全局变量.vi" "状态标记位_总磷"(w927) -> ()
              }
              frame "总氮" {
                n565 = global write "ZK非断电保存全局变量.vi" "状态标记位_总氮"(w928) -> ()
              }
              frame "CODMn" {
                n566 = global write "ZK非断电保存全局变量.vi" "状态标记位_CODMn"(w929) -> ()
              }
              frame "CODCr" {
                n567 = global write "ZK非断电保存全局变量.vi" "状态标记位_CODMn"(w930) -> ()
              }
            }
          }
          frame #1 {
            n568 = global read "ZK非断电保存全局变量.vi" "状态标记位_氨氮"() -> (w936:bool)
            n569 = global read "ZK非断电保存全局变量.vi" "状态标记位_总氮"() -> (w934:bool)
            n570 = global read "ZK非断电保存全局变量.vi" "状态标记位_CODMn"() -> (w933:bool)
            n571 = global read "ZK非断电保存全局变量.vi" "状态标记位_CODcr"() -> (w932:bool)
            n572 = global read "ZK非断电保存全局变量.vi" "状态标记位_总磷"() -> (w935:bool)
            n573 = Compound Arithmetic op=OR ("复合运算")(w936, w935, w934, w933, w932) -> (w931:bool)
            n574 = case shown="假" w931 {
              frame False {
                n575 = call "采配水启动器.vi"("启动/停止命令"=T8."停止") -> ()  [unwired: 10 in, 1 out]
              }
              frame True {
              }
            }
          }
        }
      }
      frame "判断仪器水样是否启动成功" {
        n576 = case shown="\"CODCr\"" w952 {
          tunnel: [T12."空闲" ("工作状态") w973 w975 w977 w979 w981] -> w964
          frame "null", Default {
          }
          frame "氨氮" {
            w972 = u16 3 items=["总磷"=1, "总氮"=2, "氨氮"=3, "CODMn"=21] ("站号")
            n577 = call "获取仪器仪表状态.vi"("站号"=w972) -> ("工作状态"=w973:T12)  [unwired: 10 in]
          }
          frame "总磷" {
            w974 = u16 1 items=["总磷"=1, "总氮"=2, "氨氮"=3, "CODMn"=21] ("站号")
            n578 = call "获取仪器仪表状态.vi"("站号"=w974) -> ("工作状态"=w975:T12)  [unwired: 10 in]
          }
          frame "总氮" {
            w976 = u16 2 items=["总磷"=1, "总氮"=2, "氨氮"=3, "CODMn"=21] ("站号")
            n579 = call "获取仪器仪表状态.vi"("站号"=w976) -> ("工作状态"=w977:T12)  [unwired: 10 in]
          }
          frame "CODMn" {
            w978 = u16 21 items=["总磷"=1, "总氮"=2, "氨氮"=3, "CODMn"=21] ("站号")
            n580 = call "获取仪器仪表状态.vi"("站号"=w978) -> ("工作状态"=w979:T12)  [unwired: 10 in]
          }
          frame "CODCr" {
            w980 = u16 22 items=["总磷"=1, "总氮"=2, "氨氮"=3, "CODMn"=21, "CODcr"=22] ("站号")
            n581 = call "获取仪器仪表状态.vi"("站号"=w980) -> ("工作状态"=w981:T12)  [unwired: 10 in]
          }
        }
        n582 = case shown="真" w948 {
          tunnel: w952 -> [_ w968]
          tunnel: w949 -> [_ w967]
          frame False {
          }
          frame True {
            n583 = call "启动日志.vi"("日志信息"=w967, "Slave ID"=w968) -> ()  [unwired: 9 in, 1 out]
          }
        }
        n584 = Index Array(array=w957, index=5 ("索引")) -> (element=w956:refnum<vi>)
        n585 = Greater Or Equal?(x=w951, y=60) -> (x >= y?=w944:bool)
        n586 = property class="DigNum (严格)"(reference=w956) -> ("Value"=w955:u16)  [unwired: 1 in, 2 out]
        n587 = Greater Or Equal?(x=w955, y=u16 5) -> (x >= y?=w953:bool)
        n588 = Equal?(x=w964, y=T12."空闲") -> (x = y?=w945:bool)
        n589 = And(x=w944, y=w945) -> (x .and. y?=w943:bool)
        n590 = case shown="真" w943 {
          tunnel: w952 -> [_ w970]
          frame False {
          }
          frame True {
            w969 = "水样测试启动失败" ("日志信息")
            n591 = call "启动日志.vi"("日志信息"=w969, "Slave ID"=w970) -> ()  [unwired: 9 in, 1 out]
            n592 = call "报警信息记录.vi"("报警信息"=w969, "Slave ID"=w970) -> ()  [unwired: 9 in, 1 out]
          }
        }
        n593 = Select(t="启动仪器水样测试\n判断仪器水样是否启动成功" ("State(s) In (\"\")"), s=w945, f="") -> (s? t:f=w947:string)
        n594 = Select(t=w947, s=w944, f=w949) -> (s? t:f=w946:string)
        n595 = Select(t="流程结束" ("State(s) In (\"\")"), s=w953, f=w946) -> (s? t:f=w958:string)
        n596 = call "Add State to Queue.vi"("State(s) In Front (\"\")"=w958, "State(s) In (\"\")"=w966) -> ("States Out"=w965:string)  [unwired: 13 in]
      }
      frame "判断仪器加标是否启动成功" {
        n597 = case shown="\"CODCr\"" w991 {
          tunnel: [T12."空闲" ("工作状态") w1012 w1014 w1016 w1018 w1020] -> w993
          frame "null", Default {
          }
          frame "氨氮" {
            w1011 = u16 3 items=["总磷"=1, "总氮"=2, "氨氮"=3, "CODMn"=21] ("站号")
            n598 = call "获取仪器仪表状态.vi"("站号"=w1011) -> ("工作状态"=w1012:T12)  [unwired: 10 in]
          }
          frame "总磷" {
            w1013 = u16 1 items=["总磷"=1, "总氮"=2, "氨氮"=3, "CODMn"=21] ("站号")
            n599 = call "获取仪器仪表状态.vi"("站号"=w1013) -> ("工作状态"=w1014:T12)  [unwired: 10 in]
          }
          frame "总氮" {
            w1015 = u16 2 items=["总磷"=1, "总氮"=2, "氨氮"=3, "CODMn"=21] ("站号")
            n600 = call "获取仪器仪表状态.vi"("站号"=w1015) -> ("工作状态"=w1016:T12)  [unwired: 10 in]
          }
          frame "CODMn" {
            w1017 = u16 21 items=["总磷"=1, "总氮"=2, "氨氮"=3, "CODMn"=21] ("站号")
            n601 = call "获取仪器仪表状态.vi"("站号"=w1017) -> ("工作状态"=w1018:T12)  [unwired: 10 in]
          }
          frame "CODCr" {
            w1019 = u16 22 items=["总磷"=1, "总氮"=2, "氨氮"=3, "CODMn"=21, "CODcr"=22] ("站号")
            n602 = call "获取仪器仪表状态.vi"("站号"=w1019) -> ("工作状态"=w1020:T12)  [unwired: 10 in]
          }
        }
        n603 = case shown="真" w988 {
          tunnel: w987 -> [_ w1007]
          tunnel: w991 -> [_ w1006]
          frame False {
          }
          frame True {
            n604 = call "启动日志.vi"("日志信息"=w1007, "Slave ID"=w1006) -> ()  [unwired: 9 in, 1 out]
          }
        }
        n605 = Index Array(array=w997, index=6 ("索引")) -> (element=w996:refnum<vi>)
        n606 = Greater Or Equal?(x=w990, y=60) -> (x >= y?=w983:bool)
        n607 = property class="DigNum (严格)"(reference=w996) -> ("Value"=w995:u16)  [unwired: 1 in, 2 out]
        n608 = Greater Or Equal?(x=w995, y=u16 5) -> (x >= y?=w992:bool)
        n609 = Equal?(x=w993, y=T12."空闲") -> (x = y?=w984:bool)
        n610 = And(x=w983, y=w984) -> (x .and. y?=w982:bool)
        n611 = case shown="真" w982 {
          tunnel: w991 -> [_ w1009]
          frame False {
          }
          frame True {
            w1008 = "加标回收启动失败" ("日志信息")
            n612 = call "启动日志.vi"("日志信息"=w1008, "Slave ID"=w1009) -> ()  [unwired: 9 in, 1 out]
            n613 = call "报警信息记录.vi"("报警信息"=w1008, "Slave ID"=w1009) -> ()  [unwired: 9 in, 1 out]
          }
        }
        n614 = Select(t="启动仪器加标回收测试\n判断仪器加标是否启动成功" ("State(s) In (\"\")"), s=w984, f="") -> (s? t:f=w986:string)
        n615 = Select(t=w986, s=w983, f=w987) -> (s? t:f=w985:string)
        n616 = Select(t="流程结束" ("State(s) In (\"\")"), s=w992, f=w985) -> (s? t:f=w998:string)
        n617 = call "Add State to Queue.vi"("State(s) In Front (\"\")"=w998, "State(s) In (\"\")"=w1005) -> ("States Out"=w1004:string)  [unwired: 13 in]
      }
      frame "判断仪器平行样是否启动成功" {
        n618 = case shown="\"CODCr\"" w1030 {
          tunnel: [T12."空闲" ("工作状态") w1051 w1053 w1055 w1057 w1059] -> w1032
          frame "null", Default {
          }
          frame "氨氮" {
            w1050 = u16 3 items=["总磷"=1, "总氮"=2, "氨氮"=3, "CODMn"=21] ("站号")
            n619 = call "获取仪器仪表状态.vi"("站号"=w1050) -> ("工作状态"=w1051:T12)  [unwired: 10 in]
          }
          frame "总磷" {
            w1052 = u16 1 items=["总磷"=1, "总氮"=2, "氨氮"=3, "CODMn"=21] ("站号")
            n620 = call "获取仪器仪表状态.vi"("站号"=w1052) -> ("工作状态"=w1053:T12)  [unwired: 10 in]
          }
          frame "总氮" {
            w1054 = u16 2 items=["总磷"=1, "总氮"=2, "氨氮"=3, "CODMn"=21] ("站号")
            n621 = call "获取仪器仪表状态.vi"("站号"=w1054) -> ("工作状态"=w1055:T12)  [unwired: 10 in]
          }
          frame "CODMn" {
            w1056 = u16 21 items=["总磷"=1, "总氮"=2, "氨氮"=3, "CODMn"=21] ("站号")
            n622 = call "获取仪器仪表状态.vi"("站号"=w1056) -> ("工作状态"=w1057:T12)  [unwired: 10 in]
          }
          frame "CODCr" {
            w1058 = u16 22 items=["总磷"=1, "总氮"=2, "氨氮"=3, "CODMn"=21, "CODcr"=22] ("站号")
            n623 = call "获取仪器仪表状态.vi"("站号"=w1058) -> ("工作状态"=w1059:T12)  [unwired: 10 in]
          }
        }
        n624 = case shown="真" w1026 {
          tunnel: w1030 -> [_ w1046]
          tunnel: w1027 -> [_ w1045]
          frame False {
          }
          frame True {
            n625 = call "启动日志.vi"("日志信息"=w1045, "Slave ID"=w1046) -> ()  [unwired: 9 in, 1 out]
          }
        }
        n626 = Index Array(array=w1036, index=6 ("索引")) -> (element=w1035:refnum<vi>)
        n627 = Greater Or Equal?(x=w1029, y=60) -> (x >= y?=w1022:bool)
        n628 = property class="DigNum (严格)"(reference=w1035) -> ("Value"=w1034:u16)  [unwired: 1 in, 2 out]
        n629 = Greater Or Equal?(x=w1034, y=u16 5) -> (x >= y?=w1031:bool)
        n630 = Equal?(x=w1032, y=T12."空闲") -> (x = y?=w1023:bool)
        n631 = And(x=w1022, y=w1023) -> (x .and. y?=w1021:bool)
        n632 = case shown="真" w1021 {
          tunnel: w1030 -> [_ w1048]
          frame False {
          }
          frame True {
            w1047 = "平行样启动失败" ("日志信息")
            n633 = call "启动日志.vi"("日志信息"=w1047, "Slave ID"=w1048) -> ()  [unwired: 9 in, 1 out]
            n634 = call "报警信息记录.vi"("报警信息"=w1047, "Slave ID"=w1048) -> ()  [unwired: 9 in, 1 out]
          }
        }
        n635 = Select(t="启动仪器平行样测试\n判断仪器平行样是否启动成功" ("State(s) In (\"\")"), s=w1023, f="") -> (s? t:f=w1025:string)
        n636 = Select(t=w1025, s=w1022, f=w1027) -> (s? t:f=w1024:string)
        n637 = Select(t="流程结束" ("State(s) In (\"\")"), s=w1031, f=w1024) -> (s? t:f=w1037:string)
        n638 = call "Add State to Queue.vi"("State(s) In Front (\"\")"=w1037, "State(s) In (\"\")"=w1044) -> ("States Out"=w1043:string)  [unwired: 13 in]
      }
      frame "仪器加标回收测试中", "仪器平行样测试中", "仪器水样测试中" {
        n639 = case shown="\"CODCr\"" w1066 {
          tunnel: [T12."空闲" ("工作状态") w1076 w1078 w1080 w1082 w1084] -> w1065
          frame "null", Default {
          }
          frame "氨氮" {
            w1075 = u16 3 items=["总磷"=1, "总氮"=2, "氨氮"=3, "CODMn"=21] ("站号")
            n640 = call "获取仪器仪表状态.vi"("站号"=w1075) -> ("工作状态"=w1076:T12)  [unwired: 10 in]
          }
          frame "总磷" {
            w1077 = u16 1 items=["总磷"=1, "总氮"=2, "氨氮"=3, "CODMn"=21] ("站号")
            n641 = call "获取仪器仪表状态.vi"("站号"=w1077) -> ("工作状态"=w1078:T12)  [unwired: 10 in]
          }
          frame "总氮" {
            w1079 = u16 2 items=["总磷"=1, "总氮"=2, "氨氮"=3, "CODMn"=21] ("站号")
            n642 = call "获取仪器仪表状态.vi"("站号"=w1079) -> ("工作状态"=w1080:T12)  [unwired: 10 in]
          }
          frame "CODMn" {
            w1081 = u16 21 items=["总磷"=1, "总氮"=2, "氨氮"=3, "CODMn"=21] ("站号")
            n643 = call "获取仪器仪表状态.vi"("站号"=w1081) -> ("工作状态"=w1082:T12)  [unwired: 10 in]
          }
          frame "CODCr" {
            w1083 = u16 22 items=["总磷"=1, "总氮"=2, "氨氮"=3, "CODMn"=21, "CODcr"=22] ("站号")
            n644 = call "获取仪器仪表状态.vi"("站号"=w1083) -> ("工作状态"=w1084:T12)  [unwired: 10 in]
          }
        }
        n645 = case shown="真" w1064 {
          tunnel: w1066 -> [_ w1086]
          tunnel: w1067 -> [_ w1085]
          frame False {
          }
          frame True {
            n646 = call "启动日志.vi"("日志信息"=w1085, "Slave ID"=w1086) -> ()  [unwired: 9 in, 1 out]
          }
        }
        n647 = Greater Or Equal?(x=w1063, y=30) -> (x >= y?=w1060:bool)
        n648 = Equal?(x=w1065, y=T12."空闲") -> (x = y?=w1070:bool)
        n649 = And(x=w1060, y=w1070) -> (x .and. y?=w1061:bool)
        n650 = Select(t="", s=w1061, f=w1067) -> (s? t:f=w1068:string)
        n651 = call "Add State to Queue.vi"("State(s) In Front (\"\")"=w1068, "State(s) In (\"\")"=w1073) -> ("States Out"=w1072:string)  [unwired: 13 in]
      }
    }
    n652 = Not(x=w71) -> (.not. x?=w70:bool)
    n653 = call "状态标记位读写.vi"("更新状态？"=TRUE, "Slave ID"=w69, "状态"=w70) -> ()  [unwired: 8 in, 1 out]
  }
